vi "Dashboard Main.vi"() -> ()   [LabVIEW 2016]
uses:
  <vilib>/Utility/miscctls.llb/LVRangeTypeDef.ctl
  <vilib>/Platform/TimedLoop/XDataNode/timing_clust.ctl
  <vilib>/Platform/TimedLoop/XDataNode/nitl_modes.ctl
  <vilib>/Platform/TimedLoop/XDataNode/wakeup.ctl
  <vilib>/Utility/miscctls.llb/LVRowAndColumnTypeDef.ctl
  <vilib>/event_ctls.llb/eventvkey.ctl
  <vilib>/Rock Robotics/WPI/Dashboard/WPI_DashboardLogging Global.vi
  <vilib>/Rock Robotics/Network Tables/NT Read Numeric Array.vi
  <vilib>/Rock Robotics/Network Tables/NT Write Boolean.vi
  <vilib>/platform/TimedLoop/XDataNode/XDataNode.xnode
  <vilib>/Platform/TimedLoop/XDataNode/XDNodeRunTimeDep.lvlib
panel:
  in  "Camera Settings 3":T1={"Frame Rate"=30, "Compression"=30, "Size"=1, "DB Camera Config"=FALSE} {"Frame Rate" scale=1.0..30.0; "Compression" scale=100.0..-1.0; "Size" items=["640x480", "320x240", "160x120"]}
  out "Camera Info 3":cluster{"Mbps LED":bool, "Mbps":dbl, "fps":dbl} {"fps" format="%#.1g"; "Mbps" format="%#.1g"}
  in  "Camera Name 3":string(combo)="No Camera Selection"
  in  "Camera Settings 2":T1={"Frame Rate"=30, "Compression"=30, "Size"=1, "DB Camera Config"=FALSE} {"Frame Rate" scale=1.0..30.0; "Compression" scale=100.0..-1.0; "Size" items=["640x480", "320x240", "160x120"]}
  out "Camera Info 2":cluster{"Mbps LED":bool, "Mbps":dbl, "fps":dbl} {"fps" format="%#.1g"; "Mbps" format="%#.1g"}
  in  "Camera Name 2":string(combo)="No Camera Selection"
  in  "Camera Tab":enum32{"Cam 1", "Graphs Setup", "Graphs"}(tab)
  out "Image Message":string="Timeout in Camera Communications"
  in  "Camera Settings 1":T1={"Frame Rate"=30, "Compression"=30, "Size"=1, "DB Camera Config"=FALSE} {"Frame Rate" scale=1.0..30.0; "Compression" scale=100.0..-1.0; "Size" items=["640x480", "320x240", "160x120"]}
  out "Dashboard Image 1":T2(plugin-control)
  out "Camera Info 1":cluster{"Mbps LED":bool, "Mbps":dbl, "fps":dbl} {"fps" format="%#.1g"; "Mbps" format="%#.1g"}
  in  "Camera Name 1":string(combo)="No Camera Selection"
  in  "Graph Include Filter":string[](array[string])
  in  "Graph Exclude Filter":string[](array[string])
  in  "Combo Box 8":string(combo)
  in  "Combo Box 7":string(combo)
  in  "Combo Box 6":string(combo)
  in  "Combo Box 5":string(combo)
  in  "Combo Box 4":string(combo)
  in  "Combo Box 3":string(combo)
  in  "Combo Box 2":string(combo)
  in  "Combo Box":string(combo)
  in  "Chart Update Rate Samples":i32=10
  in  "Waveform Depth Samples":i32=6000
  out "Chart 2":waveform(dbl)[](graph)
  out "Chart":waveform(dbl)[](graph)
  in  "Pause":bool
  in  "Reset":bool
  out "Samples":i32
  in  "TCP":refnum<k5>
  in  "Rec Mode":enum32{"Stop", "Record", "Playback"}(radio)
  out "Robot IP":string
  in  "Dashboard Tab":T3(tab)
  out "NT Connection":bool
  out "MotorChart R":cluster{"Numeric":dbl, "Numeric":dbl}(graph)
  out "MotorChart L":cluster{"Numeric":dbl, "Numeric":dbl}(graph)
  out "MotorSliders R":cluster{"MotorSlide1":dbl, "MotorSlide2":dbl} {"MotorSlide2" scale=-1.0..1.0 scale format="%#_2e"; "MotorSlide1" scale=-1.0..1.0 scale format="%#_2e"}
  out "MotorSliders L":cluster{"MotorSlide1":dbl, "MotorSlide2":dbl} {"MotorSlide2" scale=-1.0..1.0 scale format="%#_2e"; "MotorSlide1" scale=-1.0..1.0 scale format="%#_2e"}
  out "Gyro":dbl(knob) scale=0.0..360.0
  out "JS1 Z":dbl(slide) scale=-1.0..1.0 scale format="%#_2e"
  out "JS1 Graph":cluster{"X":dbl, "Y":dbl}[](graph)
  out "JS1 Buttons":T4
  out "JS2 Z":dbl(slide) scale=-1.0..1.0 scale format="%#_2e"
  out "JS2 Graph":cluster{"X":dbl, "Y":dbl}[](graph)
  out "JS2 Buttons":T4
  out "Mode":T5(ring)=enum."Auto Disabled"
  out "Background":bool
  in  "Get Data":bool
  in  "DB/String 9":string
  in  "DB/String 8":string
  in  "DB/String 7":string
  in  "DB/String 6":string
  in  "DB/String 5":string
  in  "DB/String 4":string
  in  "DB/String 3":string
  in  "DB/String 2":string
  in  "DB/String 1":string
  in  "DB/String 0":string
  in  "DB/Slider 0":dbl(slide) scale=0.0..5.0
  in  "DB/Slider 1":dbl(slide) scale=0.0..5.0
  in  "DB/Slider 2":dbl(slide) scale=0.0..5.0
  in  "DB/Slider 3":dbl(slide) scale=0.0..5.0
  out "DB/LED 3":bool
  out "DB/LED 2":bool
  out "DB/LED 1":bool
  out "DB/LED 0":bool
  in  "DB/Button 3":bool
  in  "DB/Button 2":bool
  in  "DB/Button 1":bool
  in  "DB/Button 0":bool caption="New Name"
  in  "Select Auto":string(combo)="Select Autonomous ..."
  in  "Select Test":string(combo)="Select Test ..."
  in  "Test Slider":dbl(slide) scale=0.0..100.0 scale format="%#_3g"
  in  "On/Off":bool caption="Solenoid"
  in  "Test Name":u16(ring) items=["Select the test to run..."]
  in  "Test Tree":string(tree)
  in  "Motor":cluster{"Value":dbl, "Enable":bool} {"Value" scale=-1.0..1.0 scale format="%#_3g"}
  out "Progress":T6 {"Test Progress" scale=0.0..100.0}
  in  "Rev/Fwd":cluster{"Forward":bool, "Reverse":bool}
  in  "Test Ring":u16(ring) items=["Monochrome", "Color"]
  out "Cmd Status":string
  in  "Execute Command":bool
  in  "Command Params":string[][](table)
  in  "Command Selection":i32(listbox)
  in  "CheckList":i32(listbox)
  out "Tree":string(tree)
  # "HW"
  # "HW"
  # "HW"
  # "Graph 1 Variable Selection"
  # "Graph 2 Variable Selection"
  # "Joysticks"
  # "Drive Motors"
  # "Front"
  # "Right"
  # "Left"
  # "Back"
  # "This tab is a great place for autonomous settings and robot-specific values.\nPlace controls and indicators inside this tab and match name to\nDashboard Variables on robot. You can also delete this comment."
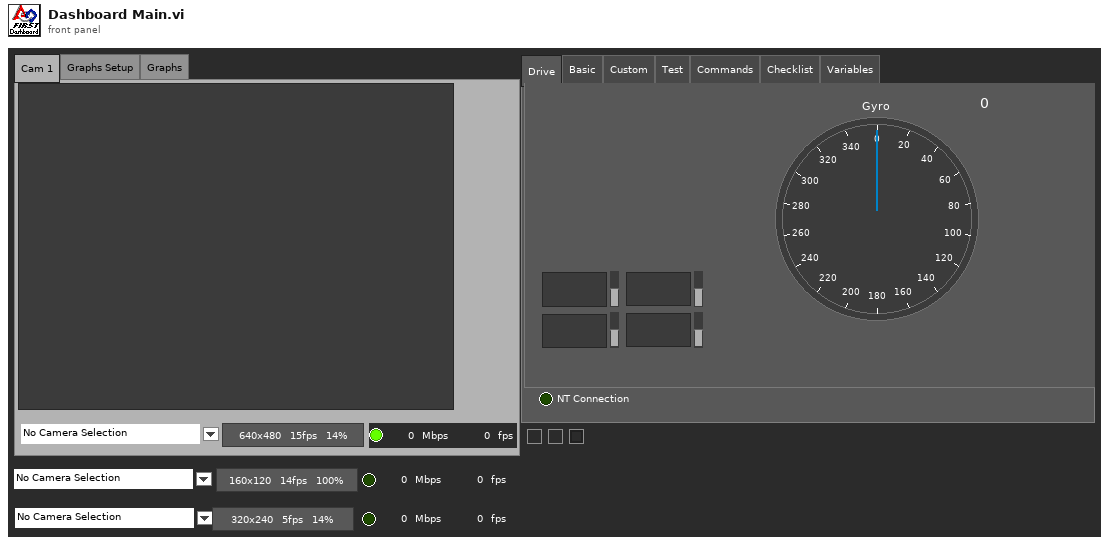
[diagram p1: front panel]
types:
  T1 = cluster{"Frame Rate":i32, "Compression":i32, "Size":u16, "DB Camera Config":bool}
  T2 = typedef "IMAQ Image.ctl" = refnum<image>
  T3 = enum32{"Drive", "Basic", "Custom", "Test", "Commands", "Checklist", "Variables"}
  T4 = cluster{bool, bool, bool, bool, bool, bool, bool, bool, bool, bool, bool, bool}
  T5 = enum8{"Tele-Op Disabled", "Tele-Op Enabled", "Auto Disabled", "Auto Enabled", "Test Disabled", "Test Enabled", "Disconnected", "No Code", "E-Stop"}
  T6 = cluster{"Test Progress":u8, "Test Progress Text":string}
  T7 = typedef "LVRangeTypeDef.ctl" = cluster{"Minimum":dbl, "Maximum":dbl, "Increment":dbl, "Minor Increment":dbl, "Start":dbl}
  T8 = cluster{"IDs":cluster{"RPC field ID":u16, "Unique ID":u16}, "String":string}
  T9 = enum32{"Drive", "Basic", "Custom", "Test", "Checklist", "Variables"}
  T10 = typedef "Image Type" = u32
  T11 = cluster{"Error Strings":string, "Disable Counts":cluster{u16, u16}, "Rail Faults":cluster{u16, u16, u16}, "Robot IP":string, "DB Mode":u8, "Event Info":cluster{"Name":string, "Type":u8, "Number":u16, "Replay":u8}}
  T12 = cluster{"Storage":cluster{"Disk Free":u64, "RAM Block":u32, "RAM free":u32}, "CPU Utilization":cluster{"CPU % ISR":sgl, "CPU % Time Crit":sgl, "CPU % Timed Str":sgl, "CPU % High":sgl, "CPU % Above":sgl, "CPU % Normal":sgl, "CPU % Low":sgl}, "CAN":cluster{"% Bus Utilization":sgl, "Bus Off Cnt":u32, "TX_FIFO Full Cnt":u32, "Receive Error Cnt":u8, "Transmit Error Cnt":u8}, "HID":cluster{"HID Outputs":u32, "Rumble Low":u16, "Rumble High":u16}[]}
  T13 = cluster{"Status bits":cluster{"Test Mode":bool, "Autonomous":bool, "Enabled":bool, "Code Start":bool, "Brownout":bool, "Reserved 2":bool, "Reserved 3":bool, "E-Stop":bool}, "Code Trace":cluster{"Disabled":bool, "TeleOp":bool, "Auto":bool, "Test":bool}, "Controller Type":enum16{"unknown", "cRIO", "roboRio"}, "Code?":enum16{"unknown", "noCode", "code"}, "Battery V":dbl}
  T14 = cluster{"Control Bits":cluster{"TestMode":bool, "Autonomous":bool, "Enabled":bool, "FMS Present":bool, bool, bool, bool, "E-Stop":bool}, "Team Station ":u8, "Countdown":sgl, "Joystick Values":cluster{"Axes":dbl[], "Buttons":bool[], "POVs":i16[]}[]}
  T15 = enum32{"Cam 1", "Cam 2", "Cam 3", "Cam 4", "Graphs Setup", "Graphs"}[]
  T16 = cluster{"Axes":dbl[], "Buttons":bool[], "POVs":i16[]}[]
  T17 = cluster{"Axes":dbl[], "Buttons":bool[], "POVs":i16[]}
  T18 = cluster{"Buttons[0]":bool, "Buttons[1]":bool, "Buttons[2]":bool, "Buttons[3]":bool, "Buttons[4]":bool, "Buttons[5]":bool, "Buttons[6]":bool, "Buttons[7]":bool, "Buttons[8]":bool, "Buttons[9]":bool, "Buttons[10]":bool, "Buttons[11]":bool}
  T19 = cluster{"Dashboard Image 1":refnum<vi>, "Dashboard Tab":refnum<vi>, "Background":refnum<vi>, "Rec Mode":refnum<vi>, "Test Slider":refnum<vi>, "On/Off ":refnum<vi>, "Test Ring":refnum<vi>, "Rev/Fwd":refnum<vi>, "Test Name":refnum<vi>, "Motor":refnum<vi>, "Progress":refnum<vi>, "CheckList":refnum<vi>, "Tree":refnum<vi>, "Test Tree":refnum<vi>, "Command Params":refnum<vi>, "Command Selection":refnum<vi>, "Execute Command":refnum<vi>, "Cmd Status":refnum<vi>, "Camera Settings 1":refnum<vi>, "Camera Name 1":refnum<vi>, "Camera Info 1":refnum<vi>, "Camera Tab":refnum<vi>, "Select Auto":refnum<vi>, "Select Test":refnum<vi>}
  T20 = cluster{"Operation":enum16{"Update", "Clear"}, "Color Box":u32}[]
  T21 = typedef "eventvkey.ctl" = enum16{"ASCII", "Enter", "Return", "Shift", "Ctrl", "Alt", "Cmd", "Opt", "Caps", "NumLock", "Clear", "Break", "Up", "Down", "Left", "Right", "Insert", "Delete", "Home", "End", "PageUp", "PageDown", "Escape", "Help", "Pause", "ScrollLock", "F1", "F2", "F3", "F4", "F5", "F6", "F7", "F8", "F9", "F10", "F11", "F12", "F13", "F14", "F15", "F16", "F17", "F18", "F19", "F20", "F21", "F22", "F23", "F24", "Play", "VolumeUp", "VolumeDown", "Mute", "Two Byte Char"}
  T22 = cluster{"Image Size":bool, "Image Type":bool, "Pixel Value":bool, "ROI Information":bool, "Zoom Factor":bool}
  T23 = cluster{"Operation":enum16{"Update", "Clear"}, "Color Box":u32}
  T24 = typedef "LVRowAndColumnTypeDef.ctl" = cluster{"Row":i32, "Column":i32}
  T25 = cluster{"Shift":bool, "Ctrl":bool, "Alt":bool, "Cmd":bool, "Opt":bool}
  T26 = typedef "XDNodeRunTimeDep.lvlib/timing_clust.ctl" = cluster{"Expected End [f-1]":u64, "Actual End [f-1]":u64, "Finished Late? [f-1]":bool, "Expected End [i-1]":u64, "Actual End [i-1]":u64, "Finished Late? [i-1]":bool, "Expected Start [i]":u64, "Actual Start [i]":u64, "Expected Start [f]":u64, "Actual Start [f]":u64, "Source Name":string, "Structure Name":string, "Period":i64, "Deadline":i64, "Offset":i64, "Start":i64, "Priority":i32, "Timeout":i32, "Mode":T27, "Wakeup Reason":T28, "Error":errorcluster, "Source Type":string, "Secondary Source Type":string, "Global End Time":u64, "Global Start Time":u64, "Frame Duration":u64, "Iteration Duration":u64, "Assigned CPU":i32, "I/O Scan Engine Mode":u32}
  T27 = typedef "XDNodeRunTimeDep.lvlib/nitl_modes.ctl" = enum32{"No Change", "Process missed periods, maintain original phase", "Discard missed periods, maintain original phase", "Process missed periods, ignore original phase", "Discard missed periods, ignore original phase"}
  T28 = typedef "XDNodeRunTimeDep.lvlib/wakeup.ctl" = enum32{"Normal", "Aborted", "Asynchronous wakeup", "Timing source error", "Timed loop error", "Timeout"}
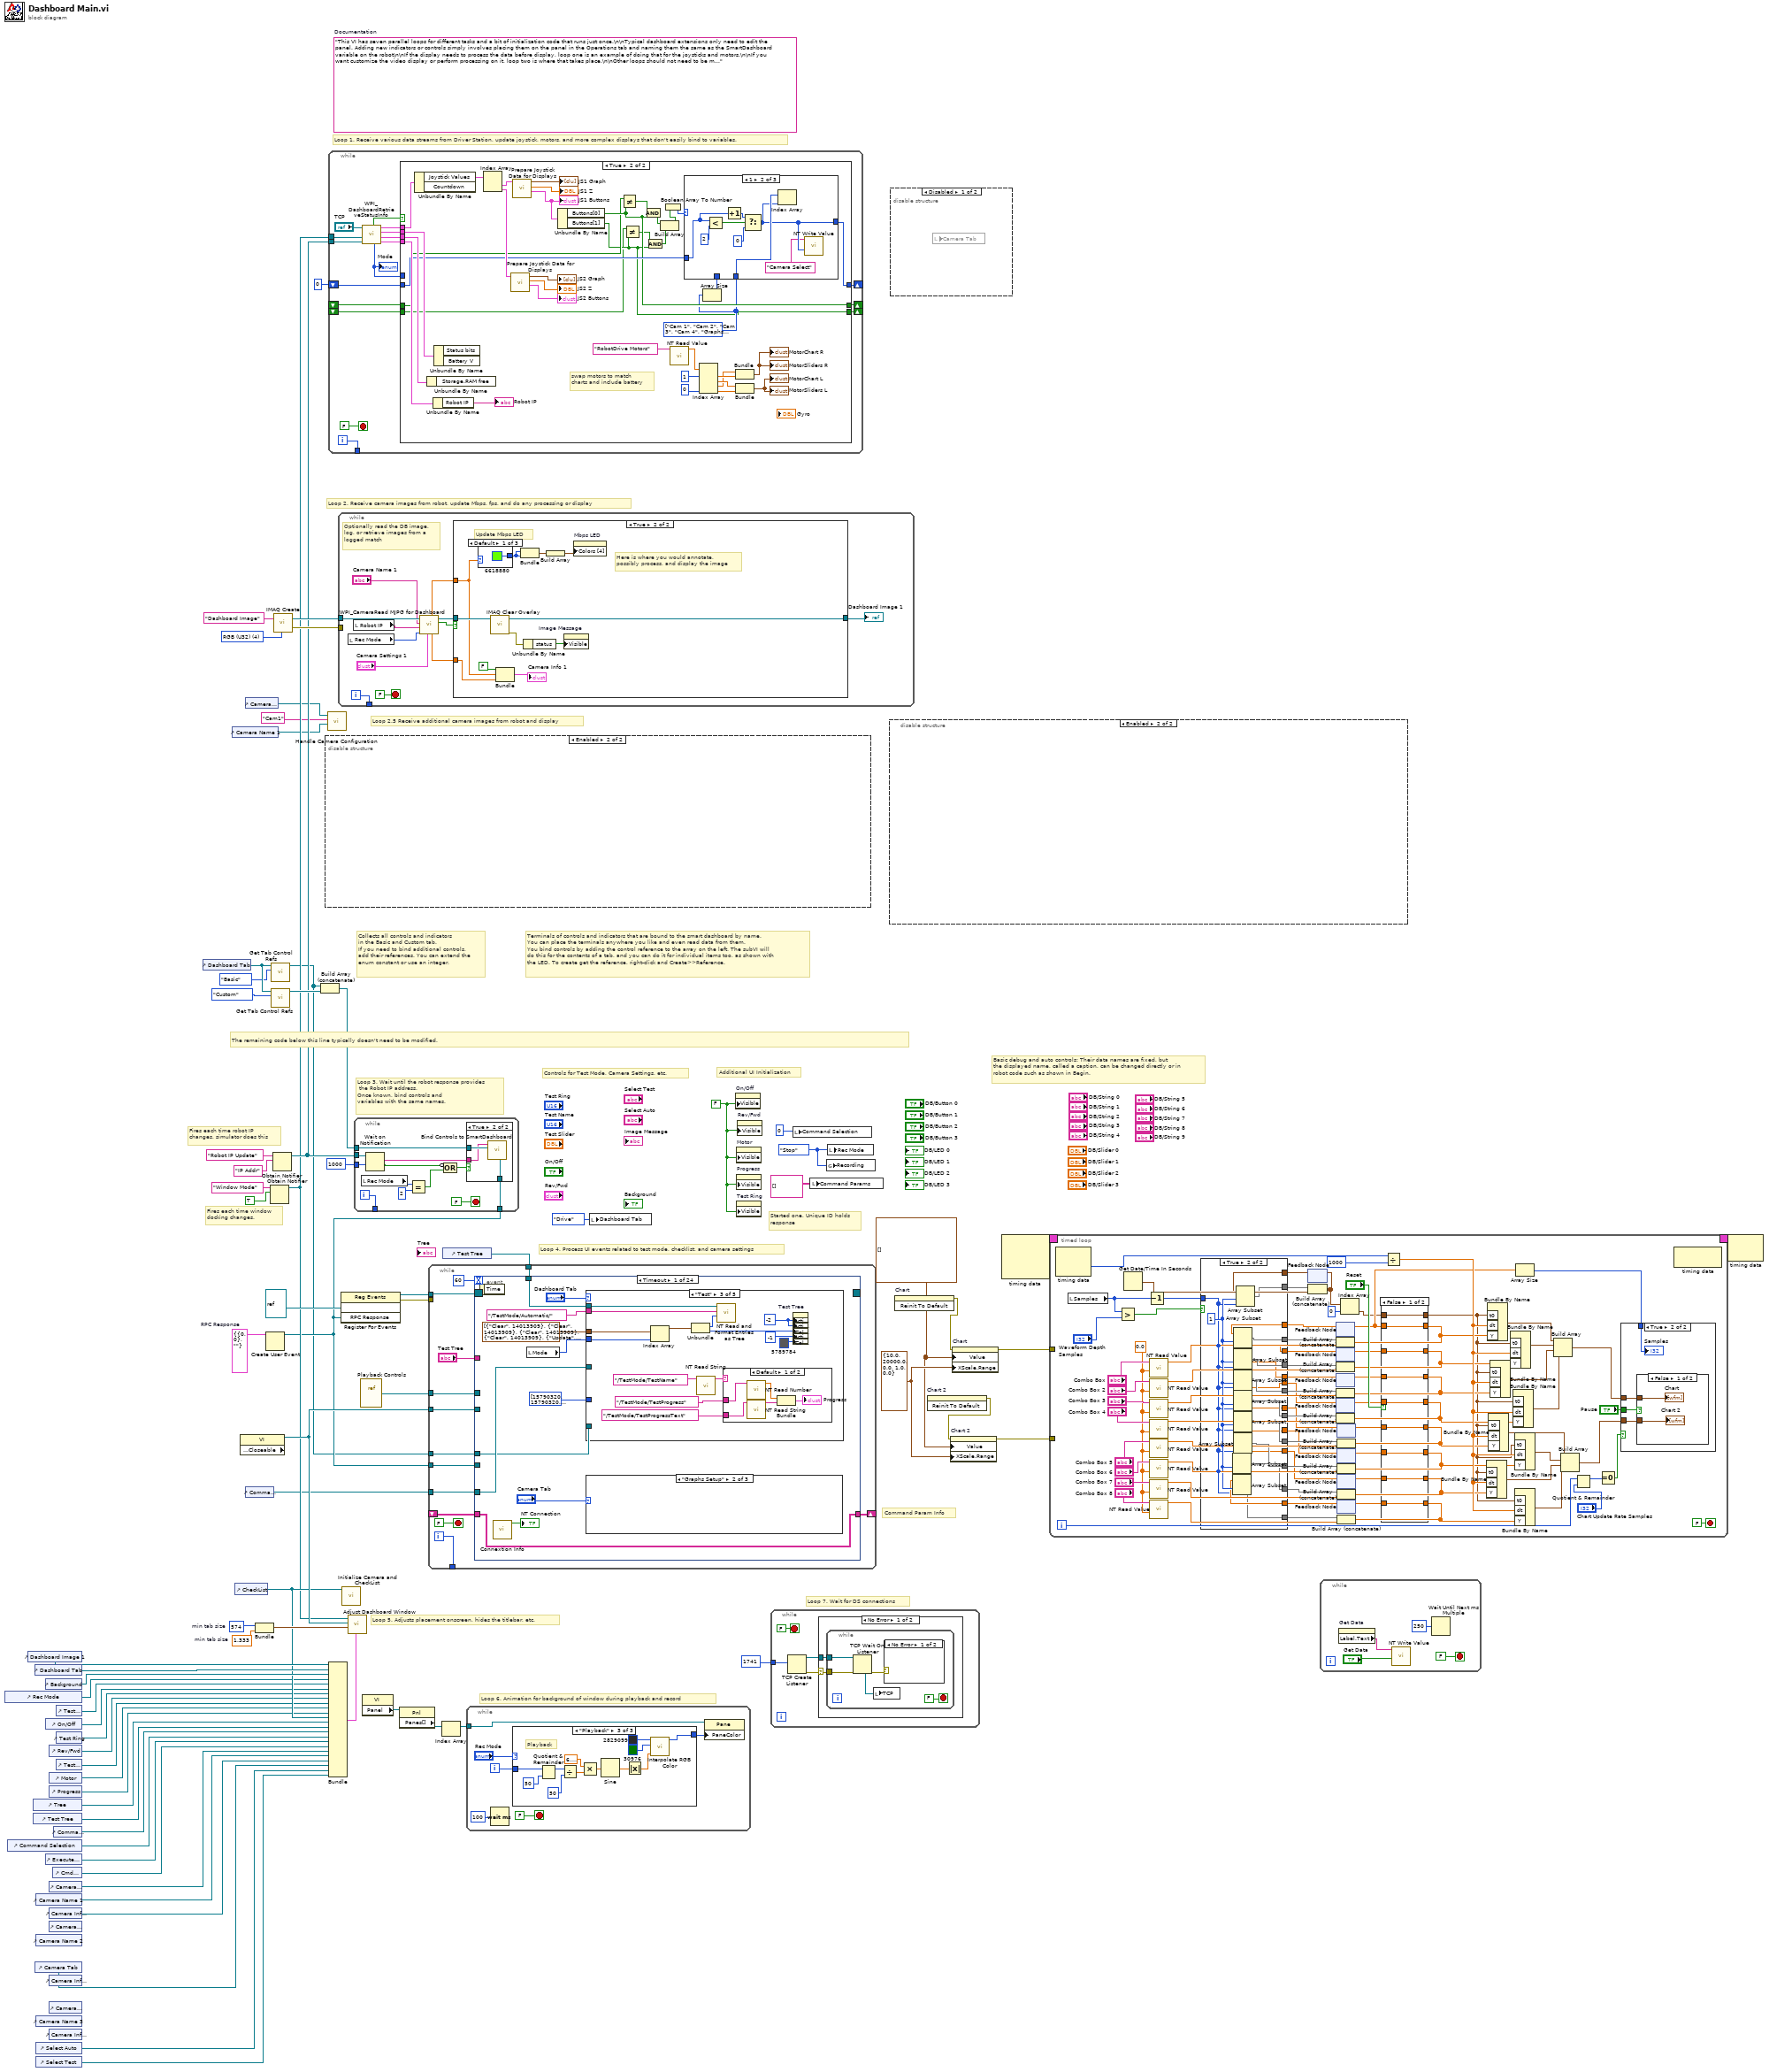
[diagram p0: block diagram]
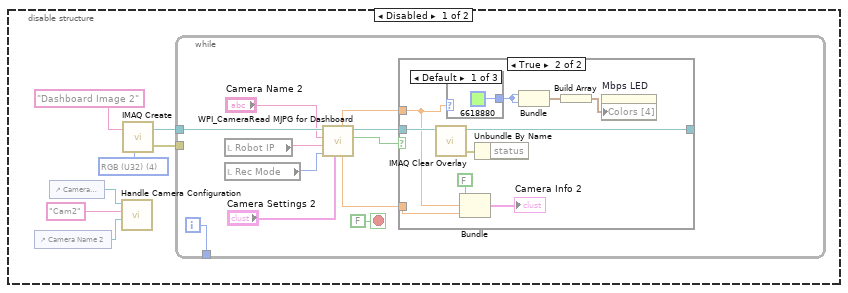
[diagram p3: hidden frame]
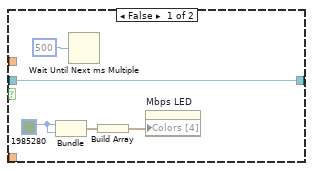
[diagram p4: hidden frame]
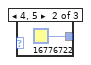
[diagram p5: hidden frame]
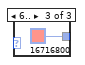
[diagram p6: hidden frame]
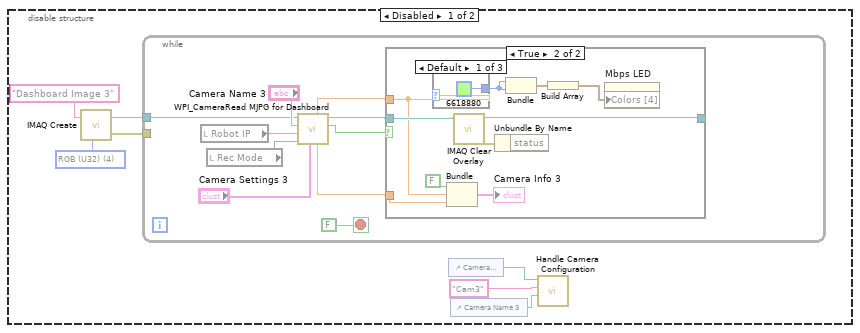
[diagram p7: hidden frame]
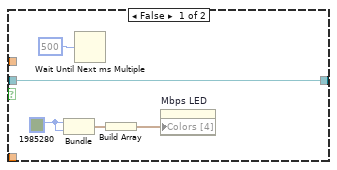
[diagram p8: hidden frame]
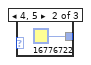
[diagram p9: hidden frame]
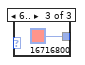
[diagram p10: hidden frame]
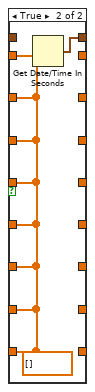
[diagram p11: hidden frame]
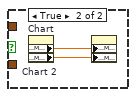
[diagram p13: hidden frame]
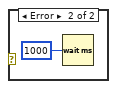
[diagram p15: hidden frame]
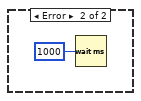
[diagram p16: hidden frame]
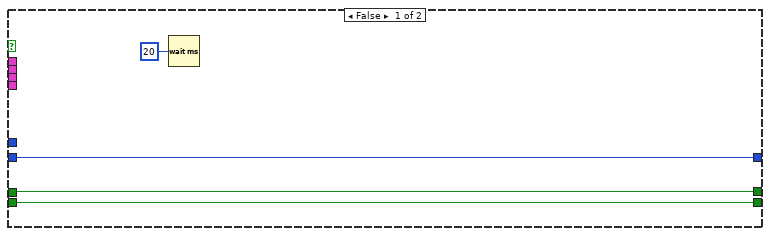
[diagram p17: hidden frame]
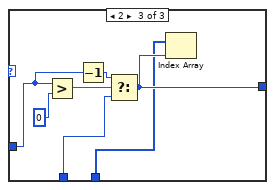
[diagram p19: hidden frame]
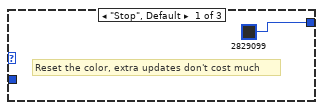
[diagram p20: hidden frame]
diagram:
  w8 = waveform(dbl)[] []
  w11 = T7 {"Minimum"=10.0, "Maximum"=20000.0, "Increment"=0.0, "Minor Increment"=1.0, "Start"=0.0} ("X Scale.Range")
  w28 = T8 {"IDs"={"RPC field ID"=0, "Unique ID"=0}, "String"=""}  # RPC Response
  w51 = 574  # min tab size
  w50 = 1.333  # min tab size
  w58 = enum32{"Stop", "Record", "Playback"}."Stop" ("Rec Mode")
  w34 = FALSE ("Visible")
  (unwired) "This VI has seven parallel loops for different tasks and a bit of initialization code that runs just once.\n\nTypical dashboard extensions only need to edit the panel. Adding new indicators or controls simply involves placing them on the panel in the Operations tab and naming them the same as the SmartDashboard variable on the robot\n\nIf the display needs to process the data before display, loop one is an example of doing that for the joysticks and motors.\n\nIf you want customize the video display or perform processing on it, loop two is where that takes place.\n\nOther loops should not need to be modified. They are pretty standard, and document the task they perform."  # Documentation
  w75 = T10 4 items=["Grayscale (U8)", "Grayscale (I16)", "Grayscale (SGL)", "Complex (CSG)", "RGB (U32)", "HSL (U32)", "RGB (U64)"] ("Image Type")
  # "Loop 2.5 Receive additional camera images from robot and display"
  # "Command Param Info"
  # "Started one, Unique ID holds\nresponse"
  # "Loop 7. Wait for DS connections"
  # "Basic debug and auto controls: Their data names are fixed, but\nthe displayed name, called a caption, can be changed directly or in\nrobot code such as shown in Begin."
  # "Controls for Test Mode, Camera Settings, etc."
  # "Additional UI Initialization"
  # "Loop 6. Animation for background of window during playback and record"
  # "Fires each time robot IP\nchanges, simulator does this"
  # "Fires each time window\ndocking changes."
  # "Collects all controls and indicators\nin the Basic and Custom tab.\nIf you need to bind additional controls,\nadd their references. You can extend the\nenum constant or use an integer."
  # "The remaining code below this line typically doesn't need to be modified."
  # "Loop 4. Process UI events related to test mode, checklist, and camera settings"
  # "Terminals of controls and indicators that are bound to the smart dashboard by name.\nYou can place the terminals anywhere you like and even read data from them.\nYou bind controls by adding the control reference to the array on the left. The subVI will\ndo this for the contents of a tab, and you can do it for individual items too, as shown with\nthe LED. To create get the reference, right-click and Create>>Reference."
  # "Loop 3. Wait until the robot response provides\n the Robot IP address.\nOnce known, bind controls and\nvariables with the same names."
  # "Loop 5. Adjusts placement onscreen, hides the titlebar, etc."
  # "Loop 1. Receive various data streams from Driver Station, update joystick, motors, and more complex displays that don't easily bind to variables."
  # "Loop 2. Receive camera images from robot, update Mbps, fps, and do any processing or display"
  n1 = control-ref of="Rec Mode"() -> (w40:refnum<vi>)
  n2 = control-ref of="Command Selection"() -> (w27:refnum<vi>)
  n3 = control-ref of="Dashboard Image 1"() -> (w53:refnum<vi>)
  n4 = control-ref of="Tree"() -> (w44:refnum<vi>)
  n5 = control-ref of="Test Tree"() -> (w43:refnum<vi>)
  n6 = control-ref of="Dashboard Tab"() -> (w52:refnum<vi>)
  n7 = control-ref of="Camera Tab"() -> (w2:refnum<vi>)
  n8 = control-ref of="Camera Name 1"() -> (w4:refnum<vi>)
  n9 = control-ref of="Camera Name 2"() -> ()  [unwired: 1 out]
  n10 = control-ref of="Camera Name 3"() -> ()  [unwired: 1 out]
  n11 = control-ref of="Select Auto"() -> (w7:refnum<vi>)
  n12 = control-ref of="Select Test"() -> (w6:refnum<vi>)
  n13 = control-ref of="Background"() -> (w48:refnum<vi>)
  n14 = control-ref of="On/Off"() -> (w38:refnum<vi>)
  n15 = control-ref of="Execute Command"() -> (w29:refnum<vi>)
  n16 = control-ref of="Rev/Fwd"() -> (w36:refnum<vi>)
  n17 = control-ref of="Motor"() -> (w41:refnum<vi>)
  n18 = control-ref of="Progress"() -> (w35:refnum<vi>)
  n19 = control-ref of="Camera Settings 1"() -> (w5:refnum<vi>)
  n20 = control-ref of="Camera Info 1"() -> (w3:refnum<vi>)
  n21 = control-ref of="Camera Settings 2"() -> ()  [unwired: 1 out]
  n22 = control-ref of="Camera Info 2"() -> ()  [unwired: 1 out]
  n23 = control-ref of="Camera Settings 3"() -> ()  [unwired: 1 out]
  n24 = control-ref of="Camera Info 3"() -> ()  [unwired: 1 out]
  n25 = control-ref of="Cmd Status"() -> (w23:refnum<vi>)
  n26 = control-ref of="Command Params"() -> (w30:refnum<vi>)
  n27 = control-ref of="Test Slider"() -> (w39:refnum<vi>)
  n28 = control-ref of="Test Ring"() -> (w37:refnum<vi>)
  n29 = control-ref of="Test Name"() -> (w42:refnum<vi>)
  n30 = control-ref of="Dashboard Tab"() -> (w56:refnum<vi>)
  n31 = control-ref of="Camera Name 1"() -> (w20:refnum<vi>)
  n32 = control-ref of="CheckList"() -> (w45:refnum<vi>)
  n33 = property class="VI" props=["Front Panel.Closeable"]() -> (reference out=w57:refnum<vi>)  [unwired: 2 in, 2 out]
  n34 = control-ref of="Camera Settings 1"() -> (w21:refnum<vi>)
  n35 = control-ref of="Command Params"() -> (w22:refnum<vi>)
  n36 = Bundle("min tab size"=w51, "min tab size"=w50) -> (w49:cluster{"min tab size":i32, "min tab size":dbl})  [unwired: 1 in]
  n37 = Create User Event(user event datatype=w28) -> (user event=w24:refnum<user-event>)  [unwired: 1 in, 1 out]
  n38 = Obtain Notifier(name (unnamed)="Window Mode", notification data type=TRUE) -> (notifier out=w32:refnum<notifier>)  [unwired: 2 in, 2 out]
  n39 = call <vilib>:"Get Tab Control Refs.vi"("Page Index"=T9."Basic" ("Dashboard Tab"), "TabControl in"=w56) -> ("ControlsOnPage"=w19:refnum<vi>[])  [unwired: 9 in]
  n40 = call <vilib>:"Get Tab Control Refs.vi"("Page Index"=T9."Custom" ("Dashboard Tab"), "TabControl in"=w56) -> ("ControlsOnPage"=w55:refnum<vi>[])  [unwired: 9 in]
  n41 = Obtain Notifier(name (unnamed)="Robot IP Update", notification data type="IP Addr" ("name (unnamed)")) -> (notifier out=w33:refnum<notifier>)  [unwired: 2 in, 2 out]
  n42 = call "IMAQ Create"("Image Name"="Dashboard Image", "Image Type"=w75) -> ("New Image"=w73:T2, "error out"=w72:errorcluster)  [unwired: 2 in, 1 out]
  n43 = Build Array (concatenate)(w19, w55) -> (w54:refnum<vi>[])
  n44 = disable-structure shown="Enabled" {
    frame Disabled {
      w77 = T10 4 items=["Grayscale (U8)", "Grayscale (I16)", "Grayscale (SGL)", "Complex (CSG)", "RGB (U32)", "HSL (U32)", "RGB (U64)", "Grayscale (U16)"] ("Image Type")
      n45 = control-ref of="Camera Name 2"() -> (w79:refnum<vi>)
      n46 = control-ref of="Camera Settings 2"() -> (w80:refnum<vi>)
      n47 = call "Handle Camera Configuration.vi"("CameraNameRef"=w79, "Camera File Name"="Cam2", "ClusterRef"=w80) -> ()  [unwired: 9 in]
      n48 = call "IMAQ Create"("Image Name"="Dashboard Image 2", "Image Type"=w77) -> ("New Image"=w76:T2, "error out"=w81:errorcluster)  [unwired: 2 in, 1 out]
      n49 = while {
        tunnel: w76 -> [w87]
        tunnel: w81 -> [_]
        tunnel: [w91] -> _
        i -> [w91]
        stop <- FALSE stop-if-true
        n50 = local read "Robot IP"() -> (w85:string)
        n51 = local read "Rec Mode"() -> (w84:enum32{"Stop", "Record", "Playback"})
        n52 = call <vilib>:"WPI_CameraRead MJPG for Dashboard.vi"("Camera Settings"="Camera Settings 2", "Rec Mode"=w84, "Robot IP"=w85, "Camera Name"="Camera Name 2", "Refnum in"=w87) -> ("Active"=w90:bool, "Refnum out"=w93:T2, "FPS"=w88:dbl, "Bandwidth (Mbps)"=w89:dbl)  [unwired: 3 in]
        n53 = case shown="True" w90 {
          tunnel: w93 -> [w97 w106]
          tunnel: w89 -> [_ w103]
          tunnel: w88 -> [_ w107]
          tunnel: [w97 w105] -> _
          frame False {
            w95 = u32 1985280 ("Color Box")
            n54 = Bundle("Color Box"=w95, "Color Box"=w95) -> (w94:cluster{"Color Box":u32, "Color Box":u32})  [unwired: 1 out]
            n55 = Wait Until Next ms Multiple(millisecond multiple=u32 500) -> ()  [unwired: 1 out]
            n56 = Build Array(w94) -> (w96:cluster{"Color Box":u32, "Color Box":u32}[])
            n57 = property on="Mbps LED" class="Bool (strict)"("Colors [4]"=w96) -> ()  [unwired: 2 in, 2 out]
          }
          frame True {
            n58 = call "IMAQ Clear Overlay"("Image"=w106) -> ("error out"=w104:errorcluster, "Image Out"=w105:T2)  [unwired: 2 in, 7 out]
            n59 = case shown="Default" w103 {
              tunnel: [u32 6618880 ("Color Box") u32 16776722 ("Color Box") u32 16716800 ("Color Box")] -> w101
              frame Default {
              }
              frame 4, 5 {
              }
              frame 6.. {
              }
            }
            n60 = Bundle(FALSE, "Bandwidth (Mbps)"=w103, "FPS"=w107) -> (→"Camera Info 2":cluster{bool, "Bandwidth (Mbps)":dbl, "FPS":dbl})  [unwired: 1 in]
            n61 = Unbundle By Name(w104) -> ()  [unwired: 1 out]
            n62 = Bundle("Color Box"=w101, "Color Box"=w101) -> (w102:cluster{"Color Box":u32, "Color Box":u32})  [unwired: 1 out]
            n63 = Build Array(w102) -> (w100:cluster{"Color Box":u32, "Color Box":u32}[])
            n64 = property on="Mbps LED" class="Bool (strict)"("Colors [4]"=w100) -> ()  [unwired: 2 in, 2 out]
          }
        }
      }
    }
    frame Enabled {
    }
  }
  n65 = call "Handle Camera Configuration.vi"("CameraNameRef"=w20, "Camera File Name"="Cam1", "ClusterRef"=w21) -> ()  [unwired: 9 in]
  n66 = while {
    tunnel: [w127] -> _
    tunnel: w33 -> [w121]
    tunnel: w32 -> [w118]
    shift-right: [w116] -> _
    shift-left: 0 ("index") -> [w117]
    shift-right: [w115] -> _
    shift-left: _ -> [w114]
    shift-right: [w113] -> _
    shift-left: _ -> [w112]
    i -> [w127]
    stop <- FALSE stop-if-true
    n67 = call <vilib>:"WPI_DashboardRetrieveStatusInfo.vi"("Binding Refnum"=w121, "Window Mode Notifier"=w118, "TCP Cnx"="TCP") -> ("Power and Errors"=w122:T11, "Robot Metrics"=w125:T12, "Status Info"=w126:T13, "Control Info"=w123:T14, "Robot Mode"=w120:T5, "Process?"=w124:bool)  [unwired: 3 in]
    "Mode" <- w120
    n68 = case shown="True" w124 {
      tunnel: w126 -> [_ w170]
      tunnel: w125 -> [_ w169]
      tunnel: w123 -> [_ w168]
      tunnel: w122 -> [_ w167]
      tunnel: w120 -> [_ _]
      tunnel: w117 -> [w131 w146]
      tunnel: [w131 w145] -> w116
      tunnel: [w130 w143] -> w115
      tunnel: w114 -> [w130 w142]
      tunnel: [w129 w138] -> w113
      tunnel: w112 -> [w129 w137]
      frame False {
        n69 = Wait (ms)(milliseconds to wait=u32 20) -> ()  [unwired: 1 out]
      }
      frame True {
        w141 = T15 [enum."Cam 1", enum."Cam 2", enum."Cam 3", enum."Cam 4", enum."Graphs Setup", enum."Graphs"] items=["Cam 1", "Cam 2", "Cam 3", "Cam 4", "Graphs Setup", "Graphs"]
        # "swap motors to match\ncharts and include battery"
        n70 = Unbundle By Name(w168) -> ("Joystick Values"=w158:T16)  [unwired: 1 out]
        n71 = Unbundle By Name(w169) -> ()  [unwired: 1 out]
        n72 = Unbundle By Name(w167) -> ("Robot IP"=→"Robot IP":string)
        n73 = Unbundle By Name(w170) -> ()  [unwired: 2 out]
        n74 = Index Array(array=w158) -> (element #1=w157:T17, element #2=w154:T17)  [unwired: 2 in]
        n75 = call "Prepare Joystick Data for Displays.vi"("Joystick Values"=w154) -> ("Buttons"=→"JS2 Buttons":T18, "Z Axis"=→"JS2 Z":dbl, "Cartesian Data"=→"JS2 Graph":cluster{"X axis":dbl, "X axis":dbl}[])  [unwired: 8 in]
        n76 = call "Prepare Joystick Data for Displays.vi"("Joystick Values"=w157) -> ("Buttons"=w147:T18, "Z Axis"=→"JS1 Z":dbl, "Cartesian Data"=→"JS1 Graph":cluster{"X axis":dbl, "X axis":dbl}[])  [unwired: 8 in]
        "JS1 Buttons" <- w147
        n77 = Unbundle By Name(w147) -> ("Buttons[0]"=w143:bool, "Buttons[1]"=w138:bool)
        n78 = Not Equal?(x=w142, y=w143) -> (x != y?=w144:bool)
        n79 = Not Equal?(x=w137, y=w138) -> (x != y?=w139:bool)
        n80 = And(x=w144, y=w143) -> (x .and. y?=w136:bool)
        n81 = And(x=w139, y=w138) -> (x .and. y?=w135:bool)
        n82 = Build Array(w136, w135) -> (w134:bool[])
        n83 = Boolean Array To Number(Boolean array=w134) -> (number=w133:u32)
        n84 = call-poly <vilib>:"NT Read Value.vi"("Name"="RobotDrive Motors") -> ("Numeric Array"=w149:dbl[])  [unwired: 9 in, 1 out]
        n85 = Index Array(array=w149, index #1=1, index #4=0) -> (element #1=w162:dbl, element #2=w163:dbl, element #3=w161:dbl, element #4=w166:dbl)  [unwired: 2 in]
        n86 = Array Size(array=w141) -> (size(s)=w140:i32)
        n87 = case shown="1" w133 {
          tunnel: w141 -> [_ w176 w183]
          tunnel: w146 -> [w171 w175 w182]
          tunnel: [w171 w174 w184] -> w145
          tunnel: w140 -> [_ _ w181]
          frame 0, Default {
          }
          frame 1 {
            n88 = Less?(x=w175, y=2) -> (x < y?=w179:bool)
            n89 = Increment(x=w175) -> (x+1=w178:i32)
            n90 = Select(t=w178, s=w179, f=0) -> (s? t:f=w174:i32)
            n91 = Index Array(array=w176, index=w174) -> ()  [unwired: 1 out]
            n92 = call-poly <vilib>:"NT Write Value.vi"("Numeric"=w174, "Name"="Camera Select") -> ()  [unwired: 9 in, 1 out]
          }
          frame 2 {
            n93 = Greater?(x=w182, y=0) -> (0:w186:bool)
            n94 = Decrement(x=w182) -> (x-1=w185:i32)
            n95 = Select(t=w185, s=w186, f=w181) -> (s? t:f=w184:i32)
            n96 = Index Array(array=w183, index=w184) -> ()  [unwired: 1 out]
          }
        }
        n97 = Bundle("Numeric"=w161, "Numeric"=w162) -> (→"MotorChart R" →"MotorSliders R":cluster{"Numeric":dbl, "Numeric":dbl})  [unwired: 1 in]
        n98 = Bundle("Numeric"=w163, "Numeric"=w166) -> (→"MotorChart L" →"MotorSliders L":cluster{"Numeric":dbl, "Numeric":dbl})  [unwired: 1 in]
      }
    }
  }
  n99 = Bundle("Dashboard Image 1"=w53, "Dashboard Tab"=w52, "Background"=w48, "Rec Mode"=w40, "Test Slider"=w39, "On/Off"=w38, "Test Ring"=w37, "Rev/Fwd"=w36, "Test Name"=w42, "Motor"=w41, "Progress"=w35, "CheckList"=w45, "Tree"=w44, "Test Tree"=w43, "Command Params"=w30, "Command Selection"=w27, "Execute Command"=w29, "Cmd Status"=w23, "Camera Settings 1"=w5, "Camera Name 1"=w4, "Camera Info 1"=w3, "Camera Tab"=w2, "Select Auto"=w7, "Select Test"=w6) -> (w1:T19)  [unwired: 1 in]
  n100 = while {
    tunnel: w73 -> [w196]
    tunnel: w72 -> [_]
    tunnel: [w197] -> _
    i -> [w197]
    stop <- FALSE stop-if-true
    # "Optionally read the DB image,\nlog, or retrieve images from a\nlogged match"
    n101 = local read "Rec Mode"() -> (w192:enum32{"Stop", "Record", "Playback"})
    n102 = local read "Robot IP"() -> (w191:string)
    n103 = call <vilib>:"WPI_CameraRead MJPG for Dashboard.vi"("Camera Settings"="Camera Settings 1", "Rec Mode"=w192, "Robot IP"=w191, "Camera Name"="Camera Name 1", "Refnum in"=w196) -> ("Active"=w194:bool, "Refnum out"=w195:T2, "FPS"=w193:dbl, "Bandwidth (Mbps)"=w190:dbl)  [unwired: 3 in]
    n104 = case shown="True" w194 {
      tunnel: w195 -> [w199 w210]
      tunnel: w190 -> [_ w207]
      tunnel: w193 -> [_ w208]
      tunnel: [w199 w204] -> w187
      frame False {
        w201 = u32 1985280 ("Color Box")
        # "Sleep for 500ms"
        n105 = Bundle("Color Box"=w201, "Color Box"=w201) -> (w202:cluster{"Color Box":u32, "Color Box":u32})  [unwired: 1 out]
        n106 = Build Array(w202) -> (w200:cluster{"Color Box":u32, "Color Box":u32}[])
        n107 = property on="Mbps LED" class="Bool (strict)"("Colors [4]"=w200) -> ()  [unwired: 2 in, 2 out]
        n108 = Wait Until Next ms Multiple(millisecond multiple=u32 500) -> ()  [unwired: 1 out]
      }
      frame True {
        # "Here is where you would annotate,\npossibly process, and display the image"
        # "Update Mbps LED"
        n109 = case shown="Default" w207 {
          tunnel: [u32 6618880 ("Color Box") u32 16776722 ("Color Box") u32 16716800 ("Color Box")] -> w211
          frame Default {
          }
          frame 4, 5 {
          }
          frame 6.. {
          }
        }
        n110 = call "IMAQ Clear Overlay"("Image"=w210) -> ("error out"=w213:errorcluster, "Image Out"=w204:T2)  [unwired: 2 in, 7 out]
        n111 = Bundle(FALSE, "Bandwidth (Mbps)"=w207, "FPS"=w208) -> (→"Camera Info 1":cluster{bool, "Bandwidth (Mbps)":dbl, "FPS":dbl})  [unwired: 1 in]
        n112 = Bundle("Color Box"=w211, "Color Box"=w211) -> (w212:cluster{"Color Box":u32, "Color Box":u32})  [unwired: 1 out]
        n113 = Unbundle By Name(w213) -> ("status"=w214:bool)
        n114 = Build Array(w212) -> (w209:cluster{"Color Box":u32, "Color Box":u32}[])
        n115 = property on="Image Message" class="Str"("Visible"=w214) -> ()  [unwired: 2 in, 2 out]
        n116 = property on="Mbps LED" class="Bool (strict)"("Colors [4]"=w209) -> ()  [unwired: 2 in, 2 out]
      }
    }
    "Dashboard Image 1" <- w187
  }
  n117 = register-events(refnum<vi> refnum, w24) -> (reference out=w62:refnum<event-registration>, error out=w61:errorcluster)  [unwired: 2 in]
  n118 = call "Initialize Camera and CheckList.vi"("ListBox in"=w45) -> ()  [unwired: 11 in]
  n119 = call "Adjust Dashboard Window.vi"("Sizing Refnums"=w1, "Size Constraints"=w49, "VI"=w57, "WIn Mode"=w32) -> ()  [unwired: 8 in]
  n120 = while {
    tunnel: w54 -> [w229]
    tunnel: w33 -> [w227]
    tunnel: [w225] -> _
    tunnel: u32 1000 ("milliseconds to wait") -> [w224]
    tunnel: w24 -> [w218]
    i -> [w225]
    stop <- FALSE stop-if-true
    n121 = local read "Rec Mode"() -> (w220:enum32{"Stop", "Record", "Playback"})
    n122 = Wait on Notification(notifier=w227, timeout in ms (-1)=w224) -> (notification=w226:string, timed out?=w222:bool)  [unwired: 2 in, 2 out]
    n123 = Equal?(x=w220, y=u16 2 ("Rec Mode")) -> (x = y?=w221:bool)
    n124 = Compound Arithmetic op=OR(invert w222, w221) -> (w223:bool)
    n125 = case shown="True" w223 {
      tunnel: w229 -> [_ w232]
      tunnel: w226 -> [_ w231]
      tunnel: w218 -> [_ w230]
      frame False {
      }
      frame True {
        n126 = call <vilib>:"Bind Controls to SmartDashboard.vi"("RPC ref"=w230, "Bound Control Refs"=w232, "Server IP Address"=w231) -> ()  [unwired: 9 in]
      }
    }
  }
  n127 = vi-ref "Playback Controls.vi"() -> (w63:refnum<vi>)
  n128 = property class="VI"() -> ("Panel"=w65:refnum<vi>)  [unwired: 2 in, 2 out]
  n129 = property class="Pnl"(reference=w65) -> ("Panes[]"=w66:refnum<vi>[])  [unwired: 1 in, 2 out]
  n130 = Index Array(array=w66) -> (element=w64:refnum<vi>)  [unwired: 1 in]
  n131 = control-ref of="Test Tree"() -> (w67:refnum<vi>)
  n132 = while {
    tunnel: [w242] -> _
    tunnel: w67 -> [w241]
    tunnel: w63 -> [w240]
    tunnel: w62 -> [w239]
    tunnel: w61 -> [_]
    tunnel: w57 -> [w238]
    tunnel: w24 -> [w237]
    tunnel: w22 -> [w236]
    shift-right: [w235] -> _
    shift-left: _ -> [w234]
    tunnel: w19 -> [w233]
    i -> [w242]
    stop <- FALSE stop-if-true
    n133 = event shown="[0] Timeout" {
      selector: w239 -> [_ _ _ _ _ _ _ _ _ _ _ _ _ _ _ _ _ _ _ _ _ _ _ _]
      dyn-events: [_ _ _ _ _ _ _ _ _ _ _ _ _ _ _ _ _ _ w506 _ _ _ _ _] -> _
      timeout: u32 60 ("milliseconds to wait") -> [_ _ _ _ _ _ _ _ _ _ _ _ _ _ _ _ _ _ _ _ _ _ _ _]
      tunnel: w241 -> [w255 _ _ _ _ _ _ _ _ _ _ _ _ _ _ _ _ _ _ _ _ _ _ _]
      tunnel: "Test Tree" -> [_ _ _ _ _ _ _ _ _ _ _ _ _ w473 w481 w483 w487 w495 _ _ _ _ _ _]
      tunnel: w240 -> [_ _ _ _ _ _ _ _ _ _ _ _ _ _ _ _ _ _ w508 _ w526 _ _ _]
      tunnel: w238 -> [_ _ _ _ _ _ _ _ _ _ _ _ _ _ _ _ _ _ w504 _ _ _ _ _]
      tunnel: w237 -> [_ _ _ _ _ _ _ _ _ _ _ _ _ _ _ _ _ _ w500 _ _ _ _ _]
      tunnel: w236 -> [w250 _ _ _ _ _ _ _ w424 _ _ _ _ _ _ _ _ _ _ _ _ _ _ _]
      tunnel: [w249 w295 w397 w402 w411 w415 w418 w421 w422 w431 w441 w448 w460 w472 w479 w482 w486 w494 w499 w521 w523 w527 w536 w570] -> w235
      tunnel: w234 -> [w249 w295 w397 w402 w411 w415 w418 w421 w422 _ _ w448 w460 w472 w479 w482 w486 w494 w499 w521 w523 w527 w536 w570]
      tunnel: w233 -> [w247 _ _ _ _ _ _ _ _ _ _ _ _ _ _ _ _ _ _ _ _ _ _ _]
      event Timeout {
        n134 = event-data() -> ()  [unwired: 1 in, 1 out]
        n135 = call <vilib>:"Connextion Info.vi"() -> ("Connected"=→"NT Connection":bool)  [unwired: 10 in, 1 out]
        n136 = local read "Mode"() -> (w252:T5)
        n137 = case shown="\"Test\"" "Dashboard Tab" {
          tunnel: w255 -> [_ _ w271 _ _]
          tunnel: "/TestMode/Automatic/" ("Name Pattern") -> [_ _ w270 _ _]
          tunnel: T20 [{"Operation"=enum."Clear", "Color Box"=14013909}, {"Operation"=enum."Clear", "Color Box"=14013909}, {"Operation"=enum."Clear", "Color Box"=14013909}, {"Operation"=enum."Clear", "Color Box"=14013909}, {"Operation"=enum."Update", "Color Box"=14013909}, {"Operation"=enum."Update", "Color Box"=16777215}, {"Operation"=enum."Clear", "Color Box"=14013909}, {"Operation"=enum."Clear", "Color Box"=14013909}, {"Operation"=enum."Clear", "Color Box"=14013909}] -> [_ _ w263 _ w288]
          tunnel: w252 -> [_ _ w262 _ w287]
          tunnel: u32[] [15790320, 15790320, 15790320, 15790320, 16777215, 16777215, 15790320, 15790320, 15790320] -> [_ _ _ _ w293]
          tunnel: w250 -> [_ _ _ _ w281]
          tunnel: w247 -> [_ w257 _ _ _]
          frame "Custom", Default {
          }
          frame "Basic" {
            n138 = call <vilib>:"WPI_DashboardUpdateNames.vi"("Controls on Tab"=w257) -> ()  [unwired: 11 in]
          }
          frame "Test" {
            w269 = -2 ("Active Item:Row Number")
            n139 = Index Array(array=w263, index=w262) -> (element=w264:T23)
            n140 = Unbundle(w264) -> ("Operation"=w265:enum16{"Update", "Clear"}, "Color Box"=w266:u32)
            n141 = call <vilib>:"NT Read String.vi"("Name"="/TestMode/TestName") -> ("String"=w260:string)  [unwired: 9 in, 1 out]
            n142 = call <vilib>:"NT Read and Format Entries as Tree.vi"("Operation"=w265, "Name Pattern"=w270, "Tree Refnum"=w271) -> ()  [unwired: 7 in, 2 out]
            n143 = case shown="Default" w260 {
              tunnel: "/TestMode/TestProgress" ("Name") -> [w273 _]
              tunnel: "/TestMode/TestProgressText" ("Name") -> [w272 _]
              frame Default {
                n144 = call <vilib>:"NT Read Number.vi"("Name"=w273) -> ("Numeric"=w274:dbl)  [unwired: 9 in, 1 out]
                n145 = call <vilib>:"NT Read String.vi"("Name"=w272) -> ("String"=w275:string)  [unwired: 9 in, 1 out]
                n146 = Bundle("Numeric"=w274, "String"=w275) -> (→"Progress":cluster{"Numeric":dbl, "String":string})  [unwired: 1 in]
              }
              frame "" {
                n147 = property on="Progress" class="Clust (strict)"("Visible"=FALSE) -> ()  [unwired: 2 in, 2 out]
                n148 = local write "Test Name"(u16 0) -> ()
              }
            }
            n149 = property on="Test Tree" class="Tree (strict)"("Active Item Row Number"=w269, "ActiveColNum"=w269, "CellBG"=w266, "Active Item Row Number"=-1 ("Active Item:Row Number"), "CellBG"=u32 5789784 ("Color Box")) -> ()  [unwired: 2 in, 2 out]
          }
          frame "Variables" {
            n150 = control-ref of="Tree"() -> (w280:refnum<vi>)
            n151 = call <vilib>:"NT Read and Format Entries as Tree.vi"("Operation"=enum16{"Update", "Clear"}."Update", "Tree Refnum"=w280) -> ()  [unwired: 8 in, 2 out]
          }
          frame "Commands" {
            w289 = u32 5789784 ("Color Box")
            w290 = T24 {"Row"=-1, "Column"=-2} ("Active Cell:Active Cell")
            w292 = T24 {"Row"=-2, "Column"=-2} ("Active Cell:Active Cell")
            n152 = Index Array(array=w293, index=w287) -> (element=w291:u32)
            n153 = Index Array(array=w288, index=w287) -> (element=w286:T23)
            n154 = Unbundle(w286) -> ("Operation"=w285:enum16{"Update", "Clear"})  [unwired: 1 out]
            n155 = local read "Command Selection"() -> (w284:i32)
            n156 = property on="Command Selection" class="MCListbox (strict)"("ActiveCell"=w292, "CellBG"=w291, "ActiveCell"=w290, "CellBG"=w289) -> ()  [unwired: 2 in, 2 out]
            n157 = call <vilib>:"WPI_DashboardUpdate RPC Info.vi"("Operation"=w285) -> ("update"=w283:bool, "commands"=w282:string[][])  [unwired: 9 in]
            n158 = property on="Command Selection" class="MCListbox (strict)"("ItemNames"=w282) -> ()  [unwired: 2 in, 2 out]
            n159 = property on="Command Params" class="Tbl (strict)"("Active Cell"=w292, "Cell BG Color"=w291, "Active Cell"=w290, "Cell BG Color"=w289) -> ()  [unwired: 2 in, 2 out]
            n160 = call <vilib>:"WPI_DashboardUpdate Command Params.vi"("Update"=w283, "NewVal"=w284, "Commands"=w282, "Param Tbl"=w281) -> ()  [unwired: 7 in, 1 out]
          }
        }
        n161 = case shown="\"Graphs Setup\"" "Camera Tab" {
          frame "Cam 1", Default {
          }
          frame "Graphs Setup" {
          }
          frame "Graphs" {
          }
        }
      }
      event "Test Tree": Value Change {
        # "Show appropriate\ncontrols"
        n162 = event-data() -> ("CtlRef"=w298:refnum<vi>, "NewVal"=w296:string)  [unwired: 1 in]
        n163 = call <vilib>:"WPI_UtilitiesGetTreeIOName.vi"("NewVal"=w296, "TreeControl in"=w298) -> ("I/O Name"=w299:string)  [unwired: 9 in]
        n164 = case shown="\"Camera\"" w299 {
          selector: w299 -> [_ w306 _ w328 w337 _]
          tunnel: w296 -> [_ _ w325 w327 _ w344]
          tunnel: cluster{string[]}[] [{["640x480", "320x240", "160x120"]}, {["Auto", "Fixed indoor", "Fixed outdoor 1", "Fixed outdoor 2", "Fixed fluorescent 1", "Fixed fluorescent 2", "Hold current"]}, {["Auto", "Flicker-free 50 Hz", "Flicker-free 60 Hz", "Hold current"]}, {["None", "Prioritize frame rate", "Prioritize image quality"]}, {["Monochrome", "Color"]}] -> [_ _ _ _ _ w343]
          frame Default {
            w301 = FALSE ("Visible")
            w300 = FALSE ("Visible")
            n165 = property on="Motor" class="Clust (strict)"("Visible"=w300) -> ()  [unwired: 2 in, 2 out]
            n166 = property on="Test Ring" class="Ring (strict)"("Visible"=w300) -> ()  [unwired: 2 in, 2 out]
            n167 = property on="Rev/Fwd" class="Clust (strict)"("Visible"=w301) -> ()  [unwired: 2 in, 2 out]
            n168 = property on="On/Off" class="Bool (strict)"("Visible"=w301) -> ()  [unwired: 2 in, 2 out]
            n169 = property on="Test Slider" class="Slide (strict)"("Visible"=w301) -> ()  [unwired: 2 in, 2 out]
          }
          frame "Analog Out", "Motor", "PWM" {
            w307 = FALSE ("Visible")
            n170 = case shown="\"Analog Out\"" w306 {
              tunnel: [1.0 ("Value") -1.0 ("Value") 0.0 ("Value")] -> w305
              tunnel: [255.0 ("Value") 1.0 ("Value") 5.0 ("Value")] -> w304
              tunnel: [128.0 ("Value") 0.0 ("Value") 0.0 ("Value")] -> w303
              tunnel: [64.0 ("Value") 0.5 ("Value") 1.0 ("Value")] -> w302
              frame "PWM" {
              }
              frame "Motor", Default {
              }
              frame "Analog Out" {
              }
            }
            n171 = property on="Motor" class="Clust (strict)"("Visible"=TRUE) -> ()  [unwired: 2 in, 2 out]
            n172 = property on="Value" class="Slide (strict)"("Value"=w303, "Scale.Minimum"=w305, "Scale.Maximum"=w304, "Scale.Increment"=w302) -> ()  [unwired: 2 in, 2 out]
            n173 = property on="On/Off" class="Bool (strict)"("Visible"=w307) -> ()  [unwired: 2 in, 2 out]
            n174 = property on="Test Slider" class="Slide (strict)"("Visible"=w307) -> ()  [unwired: 2 in, 2 out]
            n175 = property on="Test Ring" class="Ring (strict)"("Visible"=w307) -> ()  [unwired: 2 in, 2 out]
            n176 = property on="Rev/Fwd" class="Clust (strict)"("Visible"=w307) -> ()  [unwired: 2 in, 2 out]
          }
          frame "Servo" {
            w323 = FALSE ("Visible")
            n177 = call <vilib>:"NT Read Number.vi"("Name"=w325) -> ("Numeric"=w324:dbl)  [unwired: 9 in, 1 out]
            n178 = property on="Test Slider" class="Slide (strict)"("Visible"=TRUE, "Scale.Maximum"=170.0 ("Scale.Range:Maximum")) -> ()  [unwired: 2 in, 2 out]
            n179 = local write "Test Slider"(w324) -> ()
            n180 = property on="Motor" class="Clust (strict)"("Visible"=w323) -> ()  [unwired: 2 in, 2 out]
            n181 = property on="Rev/Fwd" class="Clust (strict)"("Visible"=w323) -> ()  [unwired: 2 in, 2 out]
            n182 = property on="On/Off" class="Bool (strict)"("Visible"=w323) -> ()  [unwired: 2 in, 2 out]
            n183 = property on="Test Ring" class="Ring (strict)"("Visible"=w323) -> ()  [unwired: 2 in, 2 out]
          }
          frame "Relay", "Solenoid" {
            w326 = FALSE ("Visible")
            n184 = property on="Motor" class="Clust (strict)"("Visible"=w326) -> ()  [unwired: 2 in, 2 out]
            n185 = property on="Test Slider" class="Slide (strict)"("Visible"=w326) -> ()  [unwired: 2 in, 2 out]
            n186 = Search and Replace String(input string=w327, search string="/Value  **", replace string="/Direction") -> (result string=w333:string)  [unwired: 5 in, 3 out]
            n187 = property on="Test Ring" class="Ring (strict)"("Visible"=w326) -> ()  [unwired: 2 in, 2 out]
            n188 = call <vilib>:"NT Read String.vi"("Name"=w333) -> ("String"=w331:string)  [unwired: 9 in, 1 out]
            n189 = Equal?(x="Both directions", y=w331) -> (x = y?=w329:bool)
            n190 = Not(x=w329) -> (.not. x?=w330:bool)
            n191 = property on="Rev/Fwd" class="Clust (strict)"("Visible"=w329) -> ()  [unwired: 2 in, 2 out]
            n192 = property on="On/Off" class="Bool (strict)"("Visible"=w330, "Caption.Text"=w328) -> ()  [unwired: 2 in, 2 out]
          }
          frame "Compressor", "Digital Out" {
            w336 = FALSE ("Visible")
            # "Get direction and finish"
            n193 = property on="Motor" class="Clust (strict)"("Visible"=w336) -> ()  [unwired: 2 in, 2 out]
            n194 = property on="Test Slider" class="Slide (strict)"("Visible"=w336) -> ()  [unwired: 2 in, 2 out]
            n195 = property on="Test Ring" class="Ring (strict)"("Visible"=w336) -> ()  [unwired: 2 in, 2 out]
            n196 = property on="On/Off" class="Bool (strict)"("Visible"=TRUE, "Caption.Text"=w337) -> ()  [unwired: 2 in, 2 out]
            n197 = property on="Rev/Fwd" class="Clust (strict)"("Visible"=FALSE) -> ()  [unwired: 2 in, 2 out]
          }
          frame "Camera" {
            n198 = call <vilib>:"Get Last Path Segment.vi"("String in"=w344) -> ("String out"=w345:string)  [unwired: 10 in]
            n199 = property on="On/Off" class="Bool (strict)"("Visible"=FALSE) -> ()  [unwired: 2 in, 2 out]
            n200 = property on="Motor" class="Clust (strict)"("Visible"=FALSE) -> ()  [unwired: 2 in, 2 out]
            n201 = property on="Rev/Fwd" class="Clust (strict)"("Visible"=FALSE) -> ()  [unwired: 2 in, 2 out]
            n202 = case shown="\"White Balance  **\"" w345 {
              tunnel: w344 -> [w351 w360 w369 w378 w387 _ w393]
              tunnel: w343 -> [w349 w357 w366 w375 w384 _ _]
              frame "Size  **" {
                n203 = Index Array(array=w349) -> (element=w348:cluster{string[]})  [unwired: 1 in]
                n204 = call <vilib>:"NT Read String.vi"("Name"=w351) -> ("String"=w350:string)  [unwired: 9 in, 1 out]
                n205 = Unbundle(w348) -> (w346:string[])
                n206 = Match First String(2:w346, 3:w350) -> (0:w347:i32)  [unwired: 1 out]
                n207 = property on="Test Ring" class="Ring (strict)"("Value"=w347, "Strings []"=w346) -> ()  [unwired: 2 in, 2 out]
                n208 = property on="Test Ring" class="Ring (strict)"("Visible"=TRUE) -> ()  [unwired: 2 in, 2 out]
                n209 = property on="Test Slider" class="Slide (strict)"("Visible"=FALSE) -> ()  [unwired: 2 in, 2 out]
              }
              frame "White Balance  **" {
                n210 = Index Array(array=w357, index=1) -> (element=w358:cluster{string[]})
                n211 = call <vilib>:"NT Read String.vi"("Name"=w360) -> ("String"=w359:string)  [unwired: 9 in, 1 out]
                n212 = Unbundle(w358) -> (w355:string[])
                n213 = Match First String(2:w355, 3:w359) -> (0:w354:i32)  [unwired: 1 out]
                n214 = property on="Test Ring" class="Ring (strict)"("Value"=w354, "Strings []"=w355) -> ()  [unwired: 2 in, 2 out]
                n215 = property on="Test Ring" class="Ring (strict)"("Visible"=TRUE) -> ()  [unwired: 2 in, 2 out]
                n216 = property on="Test Slider" class="Slide (strict)"("Visible"=FALSE) -> ()  [unwired: 2 in, 2 out]
              }
              frame "Exposure  **" {
                n217 = Index Array(array=w366, index=2) -> (element=w367:cluster{string[]})
                n218 = call <vilib>:"NT Read String.vi"("Name"=w369) -> ("String"=w368:string)  [unwired: 9 in, 1 out]
                n219 = Unbundle(w367) -> (w363:string[])
                n220 = Match First String(2:w363, 3:w368) -> (0:w364:i32)  [unwired: 1 out]
                n221 = property on="Test Ring" class="Ring (strict)"("Value"=w364, "Strings []"=w363) -> ()  [unwired: 2 in, 2 out]
                n222 = property on="Test Ring" class="Ring (strict)"("Visible"=TRUE) -> ()  [unwired: 2 in, 2 out]
                n223 = property on="Test Slider" class="Slide (strict)"("Visible"=FALSE) -> ()  [unwired: 2 in, 2 out]
              }
              frame "Exposure Priority  **" {
                n224 = Index Array(array=w375, index=3) -> (element=w376:cluster{string[]})
                n225 = call <vilib>:"NT Read String.vi"("Name"=w378) -> ("String"=w377:string)  [unwired: 9 in, 1 out]
                n226 = Unbundle(w376) -> (w372:string[])
                n227 = Match First String(2:w372, 3:w377) -> (0:w373:i32)  [unwired: 1 out]
                n228 = property on="Test Ring" class="Ring (strict)"("Value"=w373, "Strings []"=w372) -> ()  [unwired: 2 in, 2 out]
                n229 = property on="Test Ring" class="Ring (strict)"("Visible"=TRUE) -> ()  [unwired: 2 in, 2 out]
                n230 = property on="Test Slider" class="Slide (strict)"("Visible"=FALSE) -> ()  [unwired: 2 in, 2 out]
              }
              frame "Color Enable  **" {
                n231 = Index Array(array=w384, index=4) -> (element=w385:cluster{string[]})
                n232 = call <vilib>:"NT Read String.vi"("Name"=w387) -> ("String"=w386:string)  [unwired: 9 in, 1 out]
                n233 = Unbundle(w385) -> (w381:string[])
                n234 = Match First String(2:w381, 3:w386) -> (0:w382:i32)  [unwired: 1 out]
                n235 = property on="Test Ring" class="Ring (strict)"("Value"=w382, "Strings []"=w381) -> ()  [unwired: 2 in, 2 out]
                n236 = property on="Test Ring" class="Ring (strict)"("Visible"=TRUE) -> ()  [unwired: 2 in, 2 out]
                n237 = property on="Test Slider" class="Slide (strict)"("Visible"=FALSE) -> ()  [unwired: 2 in, 2 out]
              }
              frame Default {
                n238 = property on="Test Ring" class="Ring (strict)"("Visible"=FALSE) -> ()  [unwired: 2 in, 2 out]
                n239 = property on="Test Slider" class="Slide (strict)"("Visible"=FALSE) -> ()  [unwired: 2 in, 2 out]
              }
              frame "Brightness  **", "Color Level  **", "Compression  **", "FPS  **", "Sharpness  **" {
                n240 = call <vilib>:"NT Read Number.vi"("Name"=w393) -> ("Numeric"=w392:dbl)  [unwired: 9 in, 1 out]
                n241 = local write "Test Slider"(w392) -> ()
                n242 = property on="Test Slider" class="Slide (strict)"("Visible"=TRUE, "Scale.Maximum"=100.0 ("Scale.Range:Maximum")) -> ()  [unwired: 2 in, 2 out]
                n243 = property on="Test Ring" class="Ring (strict)"("Visible"=FALSE) -> ()  [unwired: 2 in, 2 out]
              }
            }
          }
        }
        n244 = property on="Progress" class="Clust (strict)"("Visible"=FALSE) -> ()  [unwired: 2 in, 2 out]
      }
      event "Test Name": Mouse Enter {
        # "Populate the ring with the list of tests"
        n245 = event-data() -> ()  [unwired: 1 in, 1 out]
        n246 = call <vilib>:"NT Read String Array.vi"("Name"="/TestMode/TestList") -> ("String Array"=w401:string[])  [unwired: 9 in, 1 out]
        n247 = Build Array (concatenate)("Select the test to run...", w401) -> (w400:string[])
        n248 = property on="Test Name" class="Ring (strict)"("Strings []"=w400) -> ()  [unwired: 2 in, 2 out]
      }
      event "Test Name": Value Change {
        w403 = FALSE ("Visible")
        # "Tell the robot the test name to run"
        n249 = event-data() -> ("NewVal"=w407:u16)  [unwired: 1 in]
        n250 = property on="Test Name" class="Ring (strict)"() -> ("Strings []"=w408:string[])  [unwired: 2 in, 2 out]
        n251 = local write "Progress"(T6 {"Test Progress"=0, "Test Progress Text"=""} ("Progress")) -> ()
        n252 = Index Array(array=w408, index=w407) -> (element=w406:string)
        n253 = call <vilib>:"NT Write String.vi"("String"=w406, "Name"="/TestMode/TestName") -> ()  [unwired: 9 in, 1 out]
        n254 = property on="Progress" class="Clust (strict)"("Visible"=TRUE) -> ()  [unwired: 2 in, 2 out]
        n255 = property on="Motor" class="Clust (strict)"("Visible"=w403) -> ()  [unwired: 2 in, 2 out]
        n256 = property on="Test Slider" class="Slide (strict)"("Visible"=w403) -> ()  [unwired: 2 in, 2 out]
        n257 = property on="On/Off" class="Bool (strict)"("Visible"=w403) -> ()  [unwired: 2 in, 2 out]
        n258 = property on="Rev/Fwd" class="Clust (strict)"("Visible"=w403) -> ()  [unwired: 2 in, 2 out]
        n259 = property on="Test Ring" class="Ring (strict)"("Visible"=w403) -> ()  [unwired: 2 in, 2 out]
      }
      event "Select Auto": Mouse Enter {
        # "Populate the combo box with the list of autonomous options"
        n260 = event-data() -> ()  [unwired: 1 in, 1 out]
        n261 = call <vilib>:"NT Read String Array.vi"("Name"="Auto List") -> ("String Array"=w410:string[])  [unwired: 9 in, 1 out]
        n262 = property on="Select Auto" class="CmbBox"("Strings[]"=w410) -> ()  [unwired: 2 in, 2 out]
      }
      event "Select Auto": Value Change {
        # "User modified the Auto Selection. Write to NT variable so robot knows."
        n263 = event-data() -> ("NewVal"=w413:string)  [unwired: 1 in]
        n264 = call <vilib>:"NT Write String.vi"("String"=w413, "Name"="Auto Selector") -> ()  [unwired: 9 in, 1 out]
      }
      event "Select Test": Mouse Enter {
        n265 = event-data() -> ()  [unwired: 1 in, 4 out]
        n266 = call-poly <vilib>:"NT Read Value.vi"("Name"="Test List") -> ("String Array"=w416:string[])  [unwired: 9 in, 1 out]
        n267 = property on="Select Test" class="CmbBox"("Strings[]"=w416) -> ()  [unwired: 2 in, 2 out]
      }
      event "Select Test": Value Change {
        n268 = event-data() -> ("NewVal"=w419:string)  [unwired: 1 in]
        n269 = call-poly <vilib>:"NT Write Value.vi"("String"=w419, "Name"="Test Selector") -> ()  [unwired: 9 in, 1 out]
      }
      event "Command Selection": Value Change {
        # "Get the params and show in table"
        n270 = event-data() -> ("NewVal"=w425:i32)  [unwired: 1 in]
        n271 = property on="Command Selection" class="MCListbox (strict)"() -> ("ItemNames"=w423:string[][])  [unwired: 2 in, 2 out]
        n272 = call <vilib>:"WPI_DashboardUpdate Command Params.vi"("NewVal"=w425, "Commands"=w423, "Param Tbl"=w424) -> ()  [unwired: 8 in, 1 out]
      }
      event "Execute Command": Value Change {
        # "Started one, Unique ID holds\nresponse"
        n273 = event-data() -> ()  [unwired: 1 in, 1 out]
        n274 = property on="Command Selection" class="MCListbox (strict)"() -> ("ItemNames"=w436:string[][])  [unwired: 2 in, 2 out]
        n275 = Index Array(array=w436, index (row)="Command Selection", index (col)=0) -> (element=w434:string)
        n276 = call <vilib>:"Invoke Commands.vi"("Command Params"="Command Params", "Function Name"=w434) -> ("Params"=w430:u8, "Started"=w429:bool)  [unwired: 7 in, 1 out]
        n277 = Array Subset(array="Command Params", length (row)=w430) -> (w431:string[][])  [unwired: 3 in]
        n278 = Select(t="Executing" ("Cmd Status"), s=w429, f="" ("Cmd Status")) -> (s? t:f=→"Cmd Status":string)
      }
      event "Command Selection": Double Click {
        n279 = event-data() -> ("Row"=w444:i32)  [unwired: 1 in]
        n280 = property on="Command Selection" class="MCListbox (strict)"() -> ("ItemNames"=w447:string[][])  [unwired: 2 in, 2 out]
        n281 = local read "Command Params"() -> (w443:string[][])
        n282 = Index Array(array=w447, index (row)=w444, index (col)=0) -> (element=w445:string)
        n283 = call <vilib>:"Invoke Commands.vi"("Command Params"=w443, "Function Name"=w445) -> ("Params"=w442:u8, "Started"=w437:bool)  [unwired: 7 in, 1 out]
        n284 = Array Subset(array=w443, length (row)=w442) -> (w441:string[][])  [unwired: 3 in]
        n285 = Select(t="Executing" ("Cmd Status"), s=w437, f="" ("Cmd Status")) -> (s? t:f=w438:string)
        n286 = local write "Cmd Status"(w438) -> ()
      }
      event "CheckList": Double Click {
        # "Shift clears all"
        # "Update symbols on the listbox"
        n287 = event-data() -> ("PlatMods.Shift"=w449:bool, "Row"=w451:i32)  [unwired: 1 in]
        n288 = case shown="True" w449 {
          tunnel: w451 -> [w455 _]
          tunnel: 1 -> [w454 _]
          frame False {
            n289 = property on="CheckList" class="LstBox (strict)"() -> ("Item Symbols"=w453:i32[])  [unwired: 2 in, 2 out]
            n290 = Replace Array Subset(array=w453, new element=w454, index=w455) -> (w452:i32[])
            n291 = property on="CheckList" class="LstBox (strict)"("Item Symbols"=w452) -> ()  [unwired: 2 in, 2 out]
          }
          frame True {
            w456 = 0 ("Top Row")
            n292 = property on="CheckList" class="LstBox (strict)"() -> ("Number of Rows"=w458:u32)  [unwired: 2 in, 2 out]
            n293 = Initialize Array(0, w458) -> (w457:i32[])
            n294 = property on="CheckList" class="LstBox (strict)"("Top Row"=w456, "Value"=w456, "Item Symbols"=w457) -> ()  [unwired: 2 in, 2 out]
          }
        }
      }
      event "CheckList": Key Down {
        # "Update symbols on the listbox\nLeft and right keys check and uncheck"
        n295 = event-data() -> ("VKey"=w462:T21)  [unwired: 1 in]
        n296 = case shown="\"Left\", \"Right\"" w462 {
          selector: w462 -> [w467 _]
          tunnel: eventvkey."Left" ("VKey") -> [w465 _]
          frame "Left", "Right" {
            n297 = Equal?(x=w465, y=w467) -> (x = y?=w466:bool)
            n298 = Select(t=0, s=w466, f=1) -> (s? t:f=w468:i32)
            n299 = property on="CheckList" class="LstBox (strict)"() -> ("Item Symbols"=w471:i32[])  [unwired: 2 in, 2 out]
            n300 = Replace Array Subset(array=w471, new element=w468, index="CheckList") -> (w470:i32[])
            n301 = property on="CheckList" class="LstBox (strict)"("Item Symbols"=w470) -> ()  [unwired: 2 in, 2 out]
          }
          frame Default {
          }
        }
      }
      event "Motor.Enable": Value Change {
        # "When the test mode otor enable helper is set, update that\ntree row item's value"
        n302 = event-data() -> ("NewVal"=w477:bool)  [unwired: 1 in]
        n303 = Unbundle("Motor") -> ("Value"=w476:dbl)  [unwired: 1 out]
        n304 = Select(t=w476, s=w477, f=0.0) -> (s? t:f=w474:dbl)
        n305 = call <vilib>:"NT Write Number.vi"("Numeric"=w474, "Name"=w473) -> ()  [unwired: 9 in, 1 out]
      }
      event "Test Slider": Value Change {
        # "When the test mode slider helper is set, update that\ntree row item's value"
        n306 = event-data() -> ("NewVal"=w480:dbl)  [unwired: 1 in]
        n307 = call <vilib>:"NT Write Number.vi"("Numeric"=w480, "Name"=w481) -> ()  [unwired: 9 in, 1 out]
      }
      event "On/Off": Value Change {
        # "When the test mode on/off helper value is set, update that\ntree row item's value"
        n308 = event-data() -> ("NewVal"=w485:bool)  [unwired: 1 in]
        n309 = Boolean To (0,1)(Boolean=w485) -> (0, 1=w484:i16)
        n310 = call <vilib>:"NT Write Number.vi"("Numeric"=w484, "Name"=w483) -> ()  [unwired: 9 in, 1 out]
      }
      event "Rev/Fwd": Value Change {
        # "When the test mode helper value for relays is set, update that\ntree row item's value"
        n311 = event-data() -> ("NewVal.Forward"=w493:bool, "NewVal.Reverse"=w492:bool)  [unwired: 1 in]
        n312 = Boolean To (0,1)(Boolean=w493) -> (0, 1=w489:i16)
        n313 = Boolean To (0,1)(Boolean=w492) -> (0, 1=w491:i16)
        n314 = Negate(x=w491) -> (-x=w490:i16)
        n315 = Add(x=w489, y=w490) -> (x+y=w488:i16)
        n316 = call <vilib>:"NT Write Number.vi"("Numeric"=w488, "Name"=w487) -> ()  [unwired: 9 in, 1 out]
      }
      event "Test Ring": Value Change {
        # "When a test mode helper value is selected from the ring,\nset the tree item's variable to the string value"
        n317 = event-data() -> ("NewVal"=w497:u16)  [unwired: 1 in]
        n318 = property on="Test Ring" class="Ring (strict)"() -> ("Strings []"=w498:string[])  [unwired: 2 in, 2 out]
        n319 = Index Array(array=w498, index=w497) -> (element=w496:string)
        n320 = call <vilib>:"NT Write String.vi"("String"=w496, "Name"=w495) -> ()  [unwired: 9 in, 1 out]
      }
      event "Rec Mode": Value Change {
        # "Update globals for recording mode and path to read log from.\nClear when logging and let NetworkTables set path for vision to\nuse."
        n321 = event-data() -> ("NewVal"=w509:enum32{"Stop", "Record", "Playback"})  [unwired: 1 in]
        n322 = global write "WPI_DashboardLogging Global.vi" "Logging Filename"(path "") -> ()
        n323 = global write "WPI_DashboardLogging Global.vi" "Recording"(w509) -> ()
        n324 = case shown="\"Playback\"" w509 {
          tunnel: w508 -> [_ w511 w520]
          tunnel: [_ _ w519] -> w506
          tunnel: [_ _ w518] -> _
          tunnel: w504 -> [_ _ w516]
          tunnel: cluster{i32, i32} {-250, 170} -> [_ _ w515]
          tunnel: [_ _ T22 {"Image Size"=TRUE, "Image Type"=TRUE, "Pixel Value"=TRUE, "ROI Information"=TRUE, "Zoom Factor"=FALSE} ("Image Information Shown:All Elements")] -> w502
          tunnel: [_ _ TRUE ("Zoom Factor")] -> w501
          tunnel: w500 -> [_ _ w512]
          frame Default {
          }
          frame "Stop", "Record" {
            # "Place Window too"
            n325 = invoke class="VI" method="FP.Close"(reference=w511) -> (reference out=w510:refnum<vi>)  [unwired: 2 in, 2 out]
            n326 = invoke class="VI" method="Abort VI"(reference=w510) -> ()  [unwired: 2 in, 3 out]
          }
          frame "Playback" {
            n327 = call "Open Playback Panel.vi"("Offset"=w515, "DB VI Ref"=w516, "Playback in"=w520) -> ("Playback out"=w517:refnum<vi>)  [unwired: 8 in]
            n328 = register-events(w517, w512) -> (reference out=w519:refnum<event-registration>, error out=w518:errorcluster)  [unwired: 2 in]
          }
        }
        n329 = property on="Dashboard Image 1" class="ImageControl"("Image Information Shown"=w502, "Image Information Visible"=w501) -> ()  [unwired: 2 in, 2 out]
        n330 = call <vilib>:"WPI_DashboardNT Log FieldName Cache.vi"("Operation"=enum16{"Lookup/Add", "Index", "Clear"}."Clear") -> ()  [unwired: 8 in, 3 out]
      }
      event Panel Close {
        w522 = enum32{"Stop", "Record", "Playback"}."Stop" ("Rec Mode")
        # "Playback window has been closed, abort"
        n331 = event-data() -> ()  [unwired: 1 in, 4 out]
        n332 = local write "Rec Mode"(w522) -> ()
        n333 = global write "WPI_DashboardLogging Global.vi" "Recording"(w522) -> ()
      }
      event Panel Close {
        # "Abort playback window and ourself"
        n334 = event-data() -> ()  [unwired: 1 in, 4 out]
        n335 = invoke class="VI" method="FP.Close"(reference=w526) -> (reference out=w525:refnum<vi>)  [unwired: 2 in, 2 out]
        n336 = invoke class="VI" method="Abort VI"(reference=w525) -> (error out=w524:errorcluster)  [unwired: 2 in, 2 out]
        n337 = invoke class="VI" method="Abort VI"(error in=w524) -> ()  [unwired: 2 in, 3 out]
      }
      event User Event {
        n338 = event-data() -> ("IDs"=w533:cluster{"RPC field ID":u16, "Unique ID":u16}, "String"=w532:string)  [unwired: 1 in]
        n339 = Bundle("IDs"=w533, "String"=w532) -> (w531:T8)  [unwired: 1 in]
        n340 = call <vilib>:"Retrieve RPC Response.vi"("RPC Response"=w531) -> ("Output"=w529:string[][])  [unwired: 10 in]
        n341 = Build Array (concatenate)(w527, w529) -> (w528:string[][])
        n342 = local write "Command Params"(w528) -> ()
        n343 = local write "Cmd Status"("" ("Cmd Status")) -> ()
      }
      event "Camera Tab": Mouse Enter {
        n344 = event-data() -> ()  [unwired: 1 in, 4 out]
        n345 = property on="Tree" class="Tree (strict)"() -> ("All Tags"=w534:string[])  [unwired: 2 in, 2 out]
        n346 = for {
          tunnel: w534 -> [w544] mode=indexing
          tunnel: [w544] -> w535 mode=indexing if=w542
          n347 = Empty String/Path?(string/path="Graph Include Filter") -> (empty?=w540:bool[])
          n348 = property on="Tree" class="Tree (strict)"("Active Item Tag"=w544, "ActiveColNum"=2 ("Active Cell:Active Column Number")) -> ("Cell String"=w550:string)  [unwired: 2 in, 2 out]
          n349 = And Array Elements(Boolean array=w540) -> (logical AND=w539:bool)
          n350 = case shown="False" w539 {
            selector: w539 -> [_ w561]
            tunnel: w544 -> [w554 _]
            tunnel: [w553 w561] -> w543
            tunnel: "Graph Include Filter" -> [w552 _]
            frame False {
              n351 = for {
                tunnel: [w560] -> w555 mode=indexing
                tunnel: w552 -> [w558] mode=indexing
                tunnel: w554 -> [w557]
                n352 = Match Pattern(string=w557, regular expression=w558) -> (match substring=w559:string)  [unwired: 1 in, 3 out]
                n353 = Empty String/Path?(string/path=w559) -> (empty?=w560:bool)
              }
              n354 = Not(x=w555) -> (.not. x?=w556:bool[])
              n355 = Or Array Elements(Boolean array=w556) -> (logical OR=w553:bool)
            }
            frame True {
            }
          }
          n356 = for {
            tunnel: "Graph Exclude Filter" -> [w565] mode=indexing
            tunnel: w544 -> [w563]
            tunnel: [w564] -> w546 mode=indexing
            n357 = Match Pattern(string=w563, regular expression=w565) -> (match substring=w562:string)  [unwired: 1 in, 3 out]
            n358 = Empty String/Path?(string/path=w562) -> (empty?=w564:bool)
          }
          n359 = Equal?(x="Numeric" ("y"), y=w550) -> (x = y?=w547:bool)
          n360 = And Array Elements(Boolean array=w546) -> (logical AND=w545:bool)
          n361 = Compound Arithmetic op=AND(w547, w545, w543) -> (w542:bool)
        }
        n362 = Build Array (concatenate)("Select Variable", w535) -> (w537:string[])
        n363 = property on="Combo Box" class="CmbBox"("Strings[]"=w537) -> ()  [unwired: 2 in, 2 out]
        n364 = property on="Combo Box 2" class="CmbBox"("Strings[]"=w537) -> ()  [unwired: 2 in, 2 out]
        n365 = property on="Combo Box 3" class="CmbBox"("Strings[]"=w537) -> ()  [unwired: 2 in, 2 out]
        n366 = property on="Combo Box 4" class="CmbBox"("Strings[]"=w537) -> ()  [unwired: 2 in, 2 out]
        n367 = property on="Combo Box 5" class="CmbBox"("Strings[]"=w537) -> ()  [unwired: 2 in, 2 out]
        n368 = property on="Combo Box 6" class="CmbBox"("Strings[]"=w537) -> ()  [unwired: 2 in, 2 out]
        n369 = property on="Combo Box 7" class="CmbBox"("Strings[]"=w537) -> ()  [unwired: 2 in, 2 out]
        n370 = property on="Combo Box 8" class="CmbBox"("Strings[]"=w537) -> ()  [unwired: 2 in, 2 out]
      }
      event "Tree": Double Click {
        n371 = event-data() -> ("PlatMods"=w569:T25, "Tag"=w568:string)  [unwired: 1 in]
        n372 = Unbundle(w569) -> ("Shift"=w567:bool)  [unwired: 4 out]
        n373 = Not(x=w567) -> (.not. x?=w566:bool)
        n374 = call <vilib>:"NT Update Persistence.vi"("Persistence"=w566, "Name"=w568) -> ()  [unwired: 9 in, 1 out]
      }
    }
  }
  n375 = while {
    tunnel: w64 -> [w572]
    i -> [w575]
    stop <- FALSE stop-if-true
    n376 = Wait (ms)(milliseconds to wait=u32 100) -> ()  [unwired: 1 out]
    n377 = case shown="\"Playback\"" "Rec Mode" {
      tunnel: w575 -> [_ _ w590]
      tunnel: [u32 2829099 ("Base Color") u32 11141120 ("Target Color") w579] -> w571
      frame "Stop", Default {
        # "Reset the color, extra updates don't cost much"
      }
      frame "Record" {
      }
      frame "Playback" {
        # "Playback"
        n378 = Quotient & Remainder(x=w590, y=u32 50 ("milliseconds to wait")) -> (x-y*floor(x/y)=w586:u32)  [unwired: 1 out]
        n379 = Divide(x=w586, y=u32 50 ("milliseconds to wait")) -> (x/y=w583:dbl)
        n380 = Multiply(x=6.283185307179586, y=w583) -> (x*y=w588:dbl)
        n381 = Sine(x=w588) -> (sin(x)=w587:dbl)
        n382 = Absolute Value(x=w587) -> (abs(x)=w580:dbl)
        n383 = call "Interpolate RGB Color.vi"("Proportion"=w580, "Target Color"=u32 30976, "Base Color"=u32 2829099) -> ("Result Color"=w579:u32)  [unwired: 8 in]
      }
    }
    n384 = property class="Pane"(reference=w572, "PaneColor"=w571) -> ()  [unwired: 1 in, 2 out]
  }
  n385 = local write "Dashboard Tab"(T3."Drive" ("Dashboard Tab")) -> ()
  n386 = property on="On/Off" class="Bool (strict)"("Visible"=w34) -> ()  [unwired: 2 in, 2 out]
  n387 = property on="Motor" class="Clust (strict)"("Visible"=w34) -> ()  [unwired: 2 in, 2 out]
  n388 = property on="Progress" class="Clust (strict)"("Visible"=w34) -> ()  [unwired: 2 in, 2 out]
  n389 = property on="Test Ring" class="Ring (strict)"("Visible"=w34) -> ()  [unwired: 2 in, 2 out]
  n390 = property on="Rev/Fwd" class="Clust (strict)"("Visible"=w34) -> ()  [unwired: 2 in, 2 out]
  n391 = while {
    tunnel: u16 1741 ("timeout ms (25000)") -> [w592]
    stop <- FALSE stop-if-true
    n392 = TCP Create Listener(10:w592) -> (0:w591:errorcluster, 3:w593:refnum<k5>)  [unwired: 4 in, 1 out]
    n393 = case shown="No Error" w591 {
      selector: w591 -> [w595 _]
      tunnel: w593 -> [w596 _]
      frame No Error {
        n394 = while {
          tunnel: w596 -> [w599]
          tunnel: w595 -> [w598]
          stop <- FALSE stop-if-true
          n395 = TCP Wait On Listener(8:w598, 11:w599) -> (0:w600:errorcluster, 4:w601:refnum<k5>)  [unwired: 2 in, 3 out]
          n396 = local write "TCP"(w601) -> ()
          n397 = case shown="No Error" w600 {
            frame No Error {
            }
            frame Error {
              n398 = Wait (ms)(milliseconds to wait=u32 1000) -> ()  [unwired: 1 out]
            }
          }
        }
      }
      frame Error {
        n399 = Wait (ms)(milliseconds to wait=u32 1000) -> ()  [unwired: 1 out]
      }
    }
  }
  n400 = local write "Command Selection"(u16 0 ("milliseconds to wait")) -> ()
  n401 = local write "Command Params"(string[][] [] ("Command Params")) -> ()
  n402 = global write "WPI_DashboardLogging Global.vi" "Recording"(w58) -> ()
  n403 = local write "Rec Mode"(w58) -> ()
  n404 = disable-structure shown="Enabled" {
    frame Disabled {
      w609 = T10 4 items=["Grayscale (U8)", "Grayscale (I16)", "Grayscale (SGL)", "Complex (CSG)", "RGB (U32)", "HSL (U32)", "RGB (U64)"] ("Image Type")
      n405 = call "IMAQ Create"("Image Name"="Dashboard Image 3", "Image Type"=w609) -> ("New Image"=w608:T2, "error out"=w607:errorcluster)  [unwired: 2 in, 1 out]
      n406 = while {
        tunnel: w608 -> [w617]
        tunnel: w607 -> [_]
        stop <- FALSE stop-if-true
        n407 = local read "Robot IP"() -> (w619:string)
        n408 = local read "Rec Mode"() -> (w620:enum32{"Stop", "Record", "Playback"})
        n409 = call <vilib>:"WPI_CameraRead MJPG for Dashboard.vi"("Camera Settings"="Camera Settings 3", "Rec Mode"=w620, "Robot IP"=w619, "Camera Name"="Camera Name 3", "Refnum in"=w617) -> ("Active"=w612:bool, "Refnum out"=w614:T2, "FPS"=w613:dbl, "Bandwidth (Mbps)"=w615:dbl)  [unwired: 3 in]
        n410 = case shown="True" w612 {
          tunnel: w614 -> [w624 w633]
          tunnel: w615 -> [_ w630]
          tunnel: w613 -> [_ w634]
          tunnel: [w624 w632] -> _
          frame False {
            w623 = u32 1985280 ("Color Box")
            n411 = Bundle("Color Box"=w623, "Color Box"=w623) -> (w622:cluster{"Color Box":u32, "Color Box":u32})  [unwired: 1 out]
            n412 = Wait Until Next ms Multiple(millisecond multiple=u32 500) -> ()  [unwired: 1 out]
            n413 = Build Array(w622) -> (w621:cluster{"Color Box":u32, "Color Box":u32}[])
            n414 = property on="Mbps LED" class="Bool (strict)"("Colors [4]"=w621) -> ()  [unwired: 2 in, 2 out]
          }
          frame True {
            n415 = case shown="Default" w630 {
              tunnel: [u32 6618880 ("Color Box") u32 16776722 ("Color Box") u32 16716800 ("Color Box")] -> w628
              frame Default {
              }
              frame 4, 5 {
              }
              frame 6.. {
              }
            }
            n416 = Bundle(FALSE, "Bandwidth (Mbps)"=w630, "FPS"=w634) -> (→"Camera Info 3":cluster{bool, "Bandwidth (Mbps)":dbl, "FPS":dbl})  [unwired: 1 in]
            n417 = call "IMAQ Clear Overlay"("Image"=w633) -> ("error out"=w631:errorcluster, "Image Out"=w632:T2)  [unwired: 2 in, 7 out]
            n418 = Unbundle By Name(w631) -> ()  [unwired: 1 out]
            n419 = Bundle("Color Box"=w628, "Color Box"=w628) -> (w629:cluster{"Color Box":u32, "Color Box":u32})  [unwired: 1 out]
            n420 = Build Array(w629) -> (w627:cluster{"Color Box":u32, "Color Box":u32}[])
            n421 = property on="Mbps LED" class="Bool (strict)"("Colors [4]"=w627) -> ()  [unwired: 2 in, 2 out]
          }
        }
      }
      n422 = control-ref of="Camera Settings 3"() -> (w605:refnum<vi>)
      n423 = control-ref of="Camera Name 3"() -> (w604:refnum<vi>)
      n424 = call "Handle Camera Configuration.vi"("CameraNameRef"=w604, "Camera File Name"="Cam3", "ClusterRef"=w605) -> ()  [unwired: 9 in]
    }
    frame Enabled {
    }
  }
  n425 = disable-structure shown="Disabled" {
    frame Disabled {
      n426 = local read "Camera Tab"() -> ()  [unwired: 1 in]
    }
    frame Enabled {
    }
  }
  n427 = invoke on="Chart" class="WFChart (strict)" method="Reinit To Default"() -> (error out=w10:errorcluster)  [unwired: 3 in, 2 out]
  n428 = invoke on="Chart 2" class="WFChart (strict)" method="Reinit To Default"() -> (error out=w9:errorcluster)  [unwired: 3 in, 2 out]
  n429 = property on="Chart 2" class="WFChart (strict)"(error in=w9, "Value"=w8, "XScale.Range"=w11) -> (error out=w12:errorcluster)  [unwired: 1 in, 1 out]
  n430 = property on="Chart" class="WFChart (strict)"(error in=w10, "Value"=w8, "XScale.Range"=w11) -> (error out=w13:errorcluster)  [unwired: 1 in, 1 out]
  n431 = node-c288() -> (w15:T26)  [unwired: 3 in]
  n432 = timed-loop {
    timing: w15 -> [_]
    timing-out: [_] -> w14
    tunnel: w13 -> [_]
    tunnel: w12 -> [_]
    i -> [w716]
    stop <- FALSE stop-if-true
    w704 = 0.0 ("Default Value")
    n433 = node-c288() -> (w703:i64)  [unwired: 1 in, 1 out]
    n434 = local read "Samples"() -> (w646:i32)
    n435 = Greater?(x=w646, y="Waveform Depth Samples") -> (0:w717:bool)
    n436 = Get Date/Time In Seconds() -> (seconds since 1Jan1904=w645:timestamp)
    n437 = Decrement(x=w646) -> (x-1=w701:i32)
    n438 = call-poly <vilib>:"NT Read Value.vi"("Default Value"=w704, "Name"="Combo Box") -> ("Numeric"=w700:dbl)  [unwired: 8 in, 1 out]
    n439 = call-poly <vilib>:"NT Read Value.vi"("Default Value"=w704, "Name"="Combo Box 2") -> ("Numeric"=w699:dbl)  [unwired: 8 in, 1 out]
    n440 = call-poly <vilib>:"NT Read Value.vi"("Default Value"=w704, "Name"="Combo Box 3") -> ("Numeric"=w698:dbl)  [unwired: 8 in, 1 out]
    n441 = call-poly <vilib>:"NT Read Value.vi"("Default Value"=w704, "Name"="Combo Box 4") -> ("Numeric"=w697:dbl)  [unwired: 8 in, 1 out]
    n442 = call-poly <vilib>:"NT Read Value.vi"("Default Value"=w704, "Name"="Combo Box 5") -> ("Numeric"=w696:dbl)  [unwired: 8 in, 1 out]
    n443 = call-poly <vilib>:"NT Read Value.vi"("Default Value"=w704, "Name"="Combo Box 6") -> ("Numeric"=w695:dbl)  [unwired: 8 in, 1 out]
    n444 = call-poly <vilib>:"NT Read Value.vi"("Default Value"=w704, "Name"="Combo Box 7") -> ("Numeric"=w694:dbl)  [unwired: 8 in, 1 out]
    n445 = call-poly <vilib>:"NT Read Value.vi"("Default Value"=w704, "Name"="Combo Box 8") -> ("Numeric"=w693:dbl)  [unwired: 8 in, 1 out]
    n446 = feedback #1() -> (w644:timestamp[])  [unwired: 1 in]
    n447 = feedback #2() -> (w680:dbl[])  [unwired: 1 in]
    n448 = feedback #3() -> (w678:dbl[])  [unwired: 1 in]
    n449 = feedback #4() -> (w676:dbl[])  [unwired: 1 in]
    n450 = feedback #5() -> (w674:dbl[])  [unwired: 1 in]
    n451 = feedback #6() -> (w672:dbl[])  [unwired: 1 in]
    n452 = feedback #7() -> (w670:dbl[])  [unwired: 1 in]
    n453 = feedback #8() -> (w668:dbl[])  [unwired: 1 in]
    n454 = feedback #9() -> (w666:dbl[])  [unwired: 1 in]
    n455 = case shown="True" w717 {
      tunnel: w701 -> [_ w750]
      tunnel: w680 -> [w747 w767]
      tunnel: [w747 w765] -> w679
      tunnel: w678 -> [w746 w764]
      tunnel: [w746 w763] -> w677
      tunnel: w676 -> [w745 w762]
      tunnel: [w745 w761] -> w675
      tunnel: w674 -> [w744 w760]
      tunnel: [w744 w759] -> w673
      tunnel: w672 -> [w743 w758]
      tunnel: [w743 w757] -> w671
      tunnel: w670 -> [w740 w756]
      tunnel: [w740 w755] -> w669
      tunnel: w668 -> [w741 w754]
      tunnel: [w741 w753] -> w667
      tunnel: w666 -> [w742 w752]
      tunnel: [w742 w751] -> w665
      tunnel: w644 -> [w739 w749]
      tunnel: [w739 w748] -> w643
      frame False {
      }
      frame True {
        w766 = 1 ("index")
        n456 = Array Subset(array=w754, index=w766, length=w750) -> (w753:dbl[])
        n457 = Array Subset(array=w752, index=w766, length=w750) -> (w751:dbl[])
        n458 = Array Subset(array=w762, index=w766, length=w750) -> (w761:dbl[])
        n459 = Array Subset(array=w760, index=w766, length=w750) -> (w759:dbl[])
        n460 = Array Subset(array=w758, index=w766, length=w750) -> (w757:dbl[])
        n461 = Array Subset(array=w756, index=w766, length=w750) -> (w755:dbl[])
        n462 = Array Subset(array=w767, index=w766, length=w750) -> (w765:dbl[])
        n463 = Array Subset(array=w764, index=w766, length=w750) -> (w763:dbl[])
        n464 = Array Subset(array=w749, index=w766, length=w750) -> (w748:timestamp[])
      }
    }
    n465 = Build Array (concatenate)(w643, w645) -> (w642:timestamp[])
    n466 = feedback-in #1(w642) -> ()
    n467 = Build Array (concatenate)(w679, w700) -> (w663:dbl[])
    n468 = Build Array (concatenate)(w677, w699) -> (w661:dbl[])
    n469 = Build Array (concatenate)(w675, w698) -> (w659:dbl[])
    n470 = Build Array (concatenate)(w673, w697) -> (w657:dbl[])
    n471 = Build Array (concatenate)(w671, w696) -> (w655:dbl[])
    n472 = Build Array (concatenate)(w669, w695) -> (w653:dbl[])
    n473 = Build Array (concatenate)(w667, w694) -> (w651:dbl[])
    n474 = Build Array (concatenate)(w665, w693) -> (w649:dbl[])
    n475 = Index Array(array=w642, index=0) -> (element=w640:timestamp)
    n476 = case shown="False" "Reset" {
      tunnel: [w728 w730] -> w648
      tunnel: w663 -> [w728 _]
      tunnel: [w727 w730] -> w662
      tunnel: w661 -> [w727 _]
      tunnel: w659 -> [w726 _]
      tunnel: [w726 w730] -> w660
      tunnel: [w725 w730] -> w658
      tunnel: w657 -> [w725 _]
      tunnel: [w724 w730] -> w656
      tunnel: w655 -> [w724 _]
      tunnel: [w723 w730] -> w654
      tunnel: w653 -> [w723 _]
      tunnel: [w722 w730] -> w652
      tunnel: w651 -> [w722 _]
      tunnel: [w721 w730] -> w650
      tunnel: w649 -> [w721 _]
      tunnel: w640 -> [w720 _]
      tunnel: [w720 w729] -> w647
      frame False {
      }
      frame True {
        w730 = dbl[] []
        n477 = Get Date/Time In Seconds() -> (seconds since 1Jan1904=w729:timestamp)
      }
    }
    n478 = feedback-in #2(w648) -> ()
    n479 = feedback-in #3(w662) -> ()
    n480 = feedback-in #4(w660) -> ()
    n481 = feedback-in #5(w658) -> ()
    n482 = feedback-in #6(w656) -> ()
    n483 = feedback-in #7(w654) -> ()
    n484 = feedback-in #8(w652) -> ()
    n485 = feedback-in #9(w650) -> ()
    n486 = Divide(x=w703, y=i64 1000) -> (x/y=w688:dbl)
    n487 = Bundle By Name("t0"=w647, "dt"=w688, "Y"=w651) -> (w683:waveform(dbl))  [unwired: 1 in]
    n488 = Bundle By Name("t0"=w647, "dt"=w688, "Y"=w663) -> (w692:waveform(dbl))  [unwired: 1 in]
    n489 = Bundle By Name("t0"=w647, "dt"=w688, "Y"=w655) -> (w686:waveform(dbl))  [unwired: 1 in]
    n490 = Bundle By Name("t0"=w647, "dt"=w688, "Y"=w659) -> (w689:waveform(dbl))  [unwired: 1 in]
    n491 = Bundle By Name("t0"=w647, "dt"=w688, "Y"=w661) -> (w691:waveform(dbl))  [unwired: 1 in]
    n492 = Bundle By Name("t0"=w647, "dt"=w688, "Y"=w657) -> (w690:waveform(dbl))  [unwired: 1 in]
    n493 = Bundle By Name("t0"=w647, "dt"=w688, "Y"=w653) -> (w684:waveform(dbl))  [unwired: 1 in]
    n494 = Bundle By Name("t0"=w647, "dt"=w688, "Y"=w649) -> (w685:waveform(dbl))  [unwired: 1 in]
    n495 = Array Size(array=w648) -> (size(s)=w639:i32)
    n496 = Build Array(w692, w691, w689, w690) -> (w687:waveform(dbl)[])
    n497 = Build Array(w686, w684, w683, w685) -> (w682:waveform(dbl)[])
    n498 = Quotient & Remainder(x=w716, y="Chart Update Rate Samples") -> (x-y*floor(x/y)=w715:i32)  [unwired: 1 out]
    n499 = Equal To 0?(x=w715) -> (x = 0?=w714:bool)
    n500 = case shown="True" w714 {
      tunnel: "Pause" -> [_ w734]
      tunnel: w687 -> [_ w733]
      tunnel: w682 -> [_ w732]
      tunnel: w639 -> [_ w731]
      frame False {
      }
      frame True {
        n501 = case shown="False" w734 {
          tunnel: w733 -> [w736 _]
          tunnel: w732 -> [w735 _]
          frame False {
            "Chart" <- w736
            "Chart 2" <- w735
          }
          frame True {
            n502 = property on="Chart" class="WFChart (strict)"() -> ("XScale.Minimum"=w737:dbl, "XScale.Maximum"=w738:dbl)  [unwired: 2 in, 2 out]
            n503 = property on="Chart 2" class="WFChart (strict)"("XScale.Minimum"=w737, "XScale.Maximum"=w738) -> ()  [unwired: 2 in, 2 out]
          }
        }
        "Samples" <- w731
      }
    }
    n504 = node-c288() -> ()  [unwired: 1 in, 1 out]
  }
  n505 = while {
    stop <- FALSE stop-if-true
    n506 = property on="Get Data" class="Bool (strict)"() -> ("Label.Text"=w772:string)  [unwired: 2 in, 2 out]
    n507 = call-poly <vilib>:"NT Write Value.vi"("Boolean"="Get Data", "Name"=w772) -> ()  [unwired: 9 in, 1 out]
    n508 = Wait Until Next ms Multiple(millisecond multiple=u32 250) -> ()  [unwired: 1 out]
  }
  n509 = node-c288(w14) -> ()  [unwired: 1 out]
